vi "UHR-Fleezers Control (fpga) - 11.7.1UCBMeng3.vi"() -> ()   [LabVIEW 2014]
doc: "UHR-Fleezers Instrument Control Code (fpga)"
uses:
  <vilib>/Platform/TimedLoop/XDataNode/timing_clust.ctl
  <vilib>/Platform/TimedLoop/XDataNode/nitl_modes.ctl
  <vilib>/Platform/TimedLoop/XDataNode/wakeup.ctl
  <vilib>/rvi/Emulation/niFpgaGetClockAttributes.vi
  <vilib>/rvi/Emulation/niFpgaSctlEmulationGetInTimedLoop.vi
  <vilib>/rvi/Emulation/niFpgaEmulationReportErrorSimple.vi
  <vilib>/rvi/Emulation/niFpgaProcessEmulError.vi
  <vilib>/rvi/eio/common/nirviEmuTemplateMethod_errors.vi
  <vilib>/rvi/Emulation/niFpgaCriticalErrorInLSC.vi
  <vilib>/rvi/interface/RandomDataEmulation/niFpgaRandomDataHandleErrors.vi
  <vilib>/eio/EIONode/EIONode.xnode
  <vilib>/eio/EIOMethodNode/EIOMethodNode.xnode
  <vilib>/rvi/DataTransferAndStorage/Container/XNode/niFpgaContainer.xnode
  <vilib>/rvi/interface/RandomDataEmulation/nirviRandomDataFpgaReadWriteTemplate.vi
  <vilib>/addons/control/pid/fpga.llb/XNode/niFpgaPID.xnode
  <vilib>/Platform/TimedLoop/XDataNode/XDataNode.xnode
  <vilib>/Platform/TimedLoop/XDataNode/XDNodeRunTimeDep.lvlib
panel:
  in  "Tab Control":T1(tab)=enum."Force FB"
  in  "Set 3":bool
  in  "Set 2":bool=TRUE
  in  "Set 1":bool=TRUE
  in  "Trap Pos to FIFO":bool
  in  "N of AI1 Int Acq Sets":i16=2 min=1 max=3 step=1
  out "AI Late Counter":u8
  in  "ai count":u16=400
  in  "+ phase":bool
  in  "Phase count adjustment":i16
  out "Relative phase":i16
  in  "AI to FIFO":bool
  out "BD1 Frequency Out 1":u64
  out "BD1 Frequency Out 2":u64
  out "Trap Pos FIFO Timeout":u16
  out "Trap AI FIFO Timeout":u16
  in  "Trap FIFO Set Timeout":i32
  in  "Tab Control 2":T2(tab)
  in  "RD":bool
  in  "FB1 output high":i16=3000
  in  "FB1 output low":i16
  in  "D1":i16
  in  "I1":i16=5
  in  "P1":i16=10
  in  "Swap F1 and F2":bool
  in  "Cont. Scan":bool
  in  "Abort scan":bool
  in  "Cycles per step":u64
  in  "Scan BD":bool
  in  "Number of scans":u16
  in  "Scan steps":u64
  in  "Scan freq.  increment":i64
  out "Scanning":bool
  in  "Start scan":bool
  in  "OSK Bd 1":bool
  in  "Reset Bd 1":bool
  in  "PMODE":bool
  in  "Direct RF Box \nCommunication":bool
  in  "Data BD 2":u8 format="%08b"
  in  "Data BD 1":u8 format="%08b"
  in  "Address":u8 format="%02x"
  in  "Update Data":bool
  in  "FPGA Controls\n RF Box":bool
  in  "Number Interlace Cycles":u8=2 min=1 max=3
  in  "Interlace Off Parameters":u8=1 min=1 max=3
  in  "Interlace ON/OFF":bool
  out "DIO Relative phase":i16
  in  "Phase count adjustment (DIO)":i16
  in  "+ phase (DIO)":bool
  out "DIO Late Counter":u8
  in  "DIO count 1 (ticks)":u16=400
  in  "DIO count 2 (ticks)":u16=400
  in  "DIO count 3 (ticks)":u16=400
  out "AI2 Y Sum Set 2":i16
  out "AI2 Y Sum Set 1":i16
  in  "FB Setpoint Set 1":i16 min=0 step=1
  in  "FB Reset Set 1":bool
  in  "FB On/Off Set 1":bool
  in  "FB Reset Set 2":bool
  in  "FB On/Off Set 2":bool
  in  "FB Setpoint Set 2":i16 min=0 step=1
  out "Scan I":u64
  in  "Amp switch delay":u8=5
  in  "XY phase ext loop method":bool
  in  "BD 2 Amplitude 1":u16
  in  "BD 1 Amplitude 1":u16
  in  "BD 2 Frequency 1":u64
  in  "BD 1 Frequency 1":u64
  in  "BD 2 Amplitude 2":u16
  in  "BD 1 Amplitude 2":u16
  in  "BD 2 Frequency 2":u64
  in  "BD 1 Frequency 2":u64
  in  "BD 2 Amplitude 3":u16
  in  "BD 1 Amplitude 3":u16
  in  "BD 2 Frequency 3":u64
  in  "BD 1 Frequency 3":u64
  in  "BD 1 Delay (ticks)":u8
  in  "BD 2 Delay (Ticks)":u8 caption="Count(Ticks)"
  in  "Next trap write delay (ticks)":u8 caption="Count(Ticks)"
  in  "Trap 1 osc enable":bool
  in  "Trap 2 osc enable":bool
  in  "FB2 output high":fxp<+/-,16,1>=0.999969482421875
  in  "FB2 output low":fxp<+/-,16,1>=-1.0
  in  "P2":fxp<+/-,16,8> format="%.11g"
  in  "I2":fxp<+/-,16,8>=10.0 format="%.11g"
  in  "D2":fxp<+/-,16,8> format="%.11g"
  in  "Negate Diff?":bool
  in  "Diff FB Measurement?":bool
  in  "FB Trig Integrate":u32=1
  out "TTrig?":bool
  in  "TTrig Negate Pos":bool=TRUE
  out "Trap Pos FB Int Signal":fxp<+/-,24,9> format="%.18g"
  out "Trap Pos FB Int-Norm Signal":fxp<+/-,16,1> format="%.16g"
  in  "FPGA TTrig Thresh":i64
  in  "FPGA Trap Trig":bool
  out "Trap Pos FB Action":i64
  in  "Trap Pos. FB Offset Factor":i64
  in  "Trap Pos. FB Mult Factor":i64=2
  in  "Trap Pos. FB Reset":bool
  in  "Trap Pos FB Monitor T1 or T2":bool
  in  "AI1 X Scale":u16
  in  "Trap Pos FB Int Count":u16=100
  in  "Trap Pos FB Negate Action":bool
  out "AI1 X Set 2":fxp<+/-,16,1>
  out "AI1 X Set 1":fxp<+/-,16,1>
  in  "Trap Pos. FB SP":fxp<+/-,16,1>
  in  "Force feedback":bool
  out "TTrig Sig":i64
  out "TTrig Fin Thresh":i64
  in  "1D or 2D Scan?":bool
  in  "Abort scan (MCL)":bool
  in  "MCL Scan Axis":bool
  in  "Cont. Scan (MCL)":bool
  out "Scan I (MCL)":u64
  in  "Number of scans (MCL)":u16
  out "Scanning MCL":bool
  in  "Scan steps (MCL)":u64
  in  "Cycles per step (MCL)":u64
  in  "Scan freq.  increment (MCL)":i16
  in  "Start scan (MCL)":bool
  in  "AO2":i16
  in  "AO1":i16
  out "MCL Late Counter":u8
  in  "MCL count":u32=800
  out "MCL Relative Phase":i16
  in  "Phase count adjustment (MCL)":i16
  in  "+ phase (MCL)":bool
  out "APD2 int gate":bool
  out "APD3 out state":bool
  in  "APD Gate Operating Mode":u8 max=2 step=1
  in  "Invert APD Gate":bool
  in  "APD Gate OFF Count":u16=100
  in  "APD Gate ON Count":u16=300
  out "APD 1 Gate Late Counter":u8
  out "APD 1 Gate Relative Phase":i16
  in  "Phase count adjustment (APD 1 Gate)":i16
  in  "+ phase (APD 1 Gate)":bool
  out "APD 2 Counts 0":u32
  out "APD 2 Counts 1":u32
  out "APD 1 Counts 0":u32
  out "APD 1 Counts 1":u32
  out "APD1 out state":bool
  in  "APD AO scale factor":i16=1
  in  "APD to FIFO":bool
  in  "APD Acq Rate Count":u32=20000000
  out "APD Acq Late Counter":u8
  out "APD Acq Relative Phase":i16
  in  "Phase Count Adjustment (APD Acq)":i16
  in  "+ phase (APD Acq)":bool
  in  "Phase count adjustment (APD 2 Gate)":i16
  out "APD 2 Gate Late Counter":u8
  out "APD 2 Gate Relative Phase":i16
  in  "+ phase (APD 2 Gate)":bool
  out "APD2 out state":bool
  out "APD 3 Counts 0":u32
  out "APD 3 Counts 1":u32
  out "APD 3 Gate Late Counter":u8
  in  "Phase count adjustment (APD 3 Gate)":i16
  out "APD 3 Gate Relative Phase":i16
  in  "+ phase (APD 3 Gate)":bool
  out "APD1 int gate":bool
  out "APD3 int gate":bool
  in  "D3":i16
  in  "I3":i16=5
  in  "P3":i16=10
  in  "Green Filter Flipper":bool
  in  "Green FB Count":u16=1200
  out "Green Late Counter":u8
  out "Green FB Relative Phase":i16
  in  "Phase count adjustment (Green FB)":i16=10
  in  "+ phase (Green FB)":bool
  out "Green FB Sum":i16
  in  "Green int current ON count adj":u16=150
  in  "Current Out":u16=30000
  in  "Green FB On/Off":bool
  in  "Green FB Setpoint":i16=250 min=0 step=1
  in  "Green FB Reset":bool
  in  "Operating Mode 2":u8=2 max=2 step=1
  in  "Invert GI 2":bool
  in  "Green interlace OFF count 2":u16=900
  in  "Green interlace ON count 2":u16=300
  out "GI Late Counter 2":u8
  out "GI Relative phase 2":i16
  in  "Phase count adjustment (GI) 2":i16=20
  in  "+ phase (GI) 2":bool
  in  "Green interlace OFF count":u16=100
  out "GI Relative phase":i16
  in  "Phase count adjustment (GI)":i16
  in  "+ phase (GI)":bool
  in  "Green interlace ON count":u16=300
  out "GI Late Counter":u8
  in  "Invert GI":bool
  in  "Operating Mode":u8 max=2 step=1
  in  "+ phase (RI)":bool
  out "RI Relative phase":i16
  out "RI Late Counter":u8
  in  "Red interlace ON count":u16=300
  in  "Red interlace OFF count":u16=100
  in  "Invert RI":bool
  in  "Red Laser Operating Mode":u8 max=2 step=1
  in  "Phase count adjustment (RI)":i16
  out "Red FB Intensity":i16
  in  "RI Current Out":u16=30000
  in  "Red FB On/Off":bool
  in  "D4":i16
  in  "I4":i16=5
  in  "P4":i16=10
  in  "Red FB Setpoint":i16=250 min=0 step=1
  in  "Red FB Reset":bool
  in  "RI Operating Mode 2":u8=2 max=2 step=1
  in  "Invert RI 2":bool
  in  "Phase count adjustment (BI AO)":i16=20
  in  "Blue current ON count adj (AO)":u16=150
  in  "BI Current Out":i16=30000
  in  "Blue FB On/Off":bool
  in  "D5":i16
  in  "I5":i16=5
  in  "P5":i16=10
  in  "Blue FB Setpoint":i16=250 min=0 step=1
  in  "Blue FB Reset":bool
  in  "BI Operating Mode (AO)":u8=2 max=2 step=1
  in  "Invert BI (AO)":bool
  in  "Blue OFF count (AO)":u16=900
  in  "Blue ON count (AO)":u16=300
  out "BI Late Counter (AO)":u8
  out "BI Relative phase (AO)":i16
  in  "+ phase (BI AO)":bool
  in  "Phase count adjustment (BI D)":i16
  in  "Blue Laser Operating Mode (D)":u8 max=2 step=1
  in  "Invert BI (D)":bool
  in  "Blue interlace OFF count (D)":u16=100
  in  "Blue interlace ON count (D)":u16=300
  out "Blue Late Counter (D)":u8
  out "BI Relative phase (D)":i16
  in  "+ phase (BI D)":bool
  out "Blue Intensity":i16
  # "Only one of these can be on\nat a time:"
  # "Raster Scan AOD"
  # "1 (X)"
  # "2 (Y)"
  # "IR Intensity Feedback (RF BD 1)"
  # "FB Gains Set 1"
  # "FB output range 1"
  # "False is usual, True is external loop method"
  # "Parameters if using the external RF switching loop"
  # "Parameters if using the usual internal RF switching method"
  # "FB Triggering Excitation Laser"
  # "Trap Pos. FB Gains"
  # "Trap Pos. FB Range"
  # "AO1 (Y)"
  # "2D"
  # "1D"
  # "AO2 (X)"
  # "APD AO for aligning"
  # "Detection Loop"
  # "Green fluorescent laser digital gate interlacing loop"
  # "0 Forced ON\n1 Forced OFF\n2 Interlacing"
  # "Green FB Gains"
  # "Red fluorescent laser digital gate interlacing loop"
  # "Detection Loop"
  # "0 Forced ON\n1 Forced OFF\n2 Interlacing"
  # "Analog/FB Control Loop\n(Disabled)"
  # "Digital Control Loop"
  # "Blue laser intensity reading"
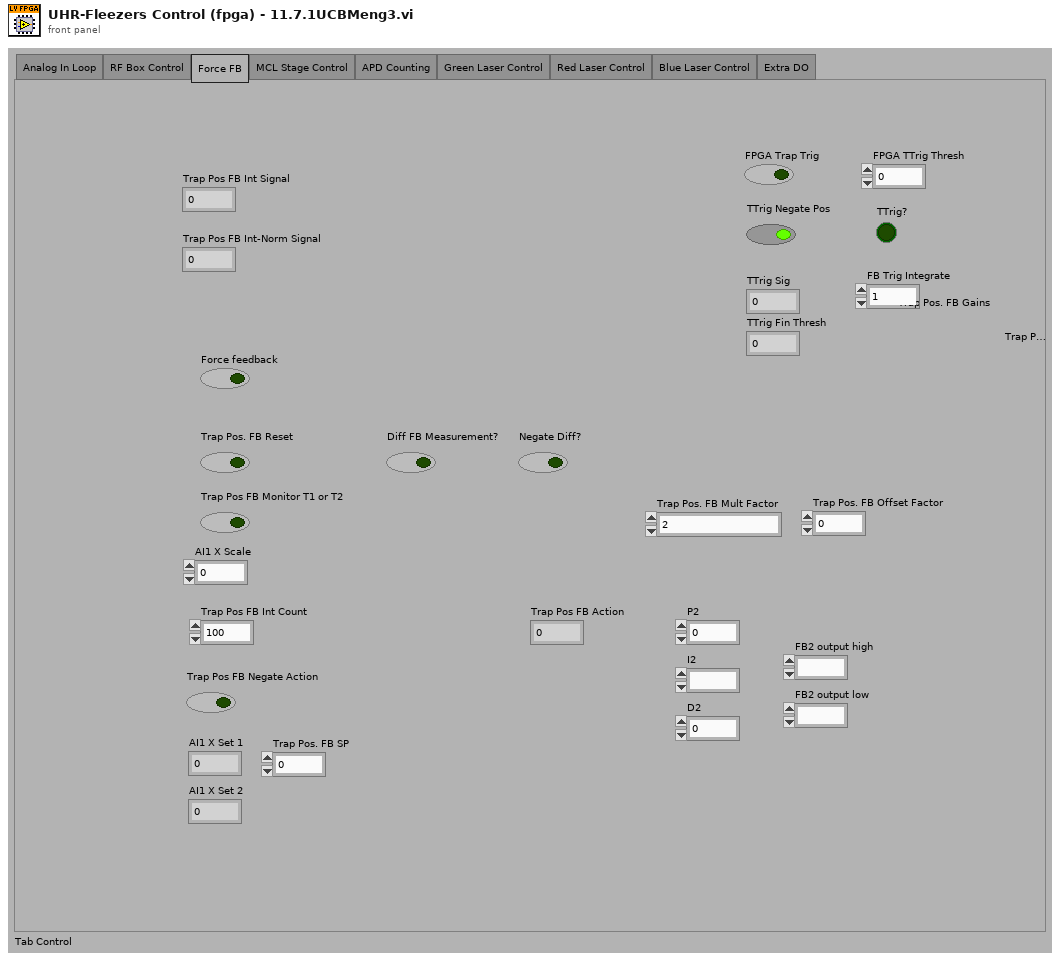
[diagram p1: front panel]
types:
  T1 = enum32{"Analog In Loop", "RF Box Control", "Force FB", "MCL Stage Control", "APD Counting", "Green Laser Control", "Red Laser Control", "Blue Laser Control", "Extra DO"}
  T2 = enum32{"Controls", "Interlacing Frequency and Amplitude Values", "Oscillate trap from memory"}
  T3 = typedef "XDNodeRunTimeDep.lvlib/timing_clust.ctl" = cluster{"Expected End [f-1]":u64, "Actual End [f-1]":u64, "Finished Late? [f-1]":bool, "Expected End [i-1]":u64, "Actual End [i-1]":u64, "Finished Late? [i-1]":bool, "Expected Start [i]":u64, "Actual Start [i]":u64, "Expected Start [f]":u64, "Actual Start [f]":u64, "Source Name":string, "Structure Name":string, "Period":i64, "Deadline":i64, "Offset":i64, "Start":i64, "Priority":i32, "Timeout":i32, "Mode":T4, "Wakeup Reason":T5, "Error":errorcluster, "Source Type":string, "Secondary Source Type":string, "Global End Time":u64, "Global Start Time":u64, "Frame Duration":u64, "Iteration Duration":u64, "Assigned CPU":i32, "I/O Scan Engine Mode":u32}
  T4 = typedef "XDNodeRunTimeDep.lvlib/nitl_modes.ctl" = enum32{"No Change", "Process missed periods, maintain original phase", "Discard missed periods, maintain original phase", "Process missed periods, ignore original phase", "Discard missed periods, ignore original phase"}
  T5 = typedef "XDNodeRunTimeDep.lvlib/wakeup.ctl" = enum32{"Normal", "Aborted", "Asynchronous wakeup", "Timing source error", "Timed loop error", "Timeout"}
  T6 = cluster{"proportional gain (Kc)":i16, "integral gain (Kc*Ts/Ti)":i16, "derivative gain (Kc*Td/Ts)":i16}
  T7 = cluster{"FB1 output high":i16, "FB1 output low":i16}
  T8 = cluster{"P2":fxp<+/-,16,8>, "I2":fxp<+/-,16,8>, "D2":fxp<+/-,16,8>}
  T9 = cluster{"FB2 output high":fxp<+/-,16,1>, "FB2 output low":fxp<+/-,16,1>}
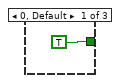
[diagram p3: hidden frame]
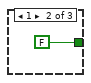
[diagram p4: hidden frame]
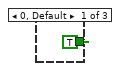
[diagram p5: hidden frame]
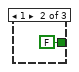
[diagram p6: hidden frame]
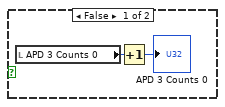
[diagram p8: hidden frame]
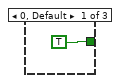
[diagram p9: hidden frame]
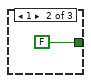
[diagram p10: hidden frame]
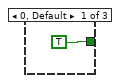
[diagram p11: hidden frame]
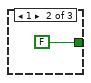
[diagram p12: hidden frame]
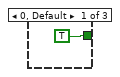
[diagram p13: hidden frame]
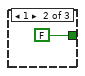
[diagram p14: hidden frame]
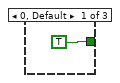
[diagram p15: hidden frame]
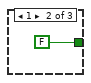
[diagram p16: hidden frame]
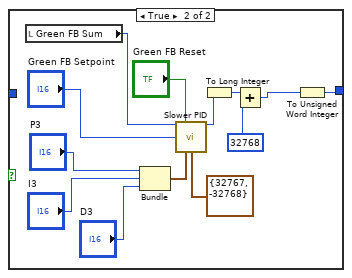
[diagram p18: hidden frame]
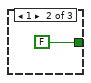
[diagram p19: hidden frame]
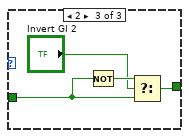
[diagram p20: hidden frame]
diagram:
  w3 = u16 0
  w5 = FALSE
  w2 = FALSE
  # "timing array current index"
  # "timing array"
  # "timing counter (phase adjusted here)"
  # "late counter"
  n1 = flat-sequence "FPGA initialization to do before running any of the loops" {
    tunnel: [u16 0 ("DIO count 3 (ticks)")] -> w1
    tunnel: [w13] -> _
    frame #0 {
      w12 = FALSE ("Enable")
      # "BD 2 (Y)"
      # "BD 1 (X)"
      # "Start up expansion chassis early\nto avoid delays later"
      # "This pin controls udclk on the RF boards.\nWhen initially configuring the boards, this pin needs to be\nconfigured as a high impedance input.  Later it will be switched\nto an output."
      # "Initial setting of DIO data and \naddress to low (before reset).  \nThis needs to happen before the other\ncontrol method loops execute."
      n2 = xnode "FPGA I/O Node"("Chassis2/Mod1/AO0"=u16 0 ("Chassis2/Mod4/AO0")) -> ("Chassis2/Mod2/AI0"=w13:i16)  [unwired: 2 in, 2 out]
      n3 = xnode "FPGA I/O Method Node"("Enable"=w12) -> ()  [unwired: 1 in, 1 out]
      n4 = xnode "FPGA I/O Method Node"("Enable"=w12) -> ()  [unwired: 1 in, 1 out]
      n5 = xnode "FPGA I/O Node"("Connector1/DIO0"=FALSE, "Connector1/DIO1"=FALSE, "Connector1/DIO2"=FALSE, "Connector1/DIO3"=FALSE, "Connector1/DIO4"=FALSE, "Connector1/DIO5"=FALSE, "Connector1/DIO6"=FALSE, "Connector1/DIO7"=FALSE, "Connector1/DIO8"=FALSE, "Connector1/DIO9"=FALSE, "Connector1/DIO10"=FALSE, "Connector1/DIO11"=FALSE, "Connector1/DIO12"=FALSE, "Connector1/DIO13"=FALSE, "Connector1/DIO15"=FALSE, "Connector1/DIO20"=FALSE, "Connector1/DIO21"=FALSE, "Connector1/DIO22"=FALSE, "Connector1/DIO23"=FALSE, "Connector1/DIO24"=FALSE, "Connector1/DIO25"=FALSE, "Connector1/DIO26"=FALSE, "Connector1/DIO27"=FALSE, "Connector1/DIO14"=FALSE) -> ()  [unwired: 24 in, 24 out]
    }
  }
  n6 = local read "AO1"() -> (w10:i16)
  n7 = local read "AO2"() -> (w9:i16)
  n8 = node-c288() -> (w8:T3)  [unwired: 1 in]
  n9 = To Unsigned Long Integer(number=w1) -> (unsigned 32bit integer=w6:u32)
  n10 = timed-loop "RF box board DIO control: control bits" {
    timing: w8 -> [_]
    timing-out: [_] -> w7
    tunnel: [w42] -> _
    tunnel: w1 -> [w42]
    stop <- FALSE stop-if-true
    n11 = xnode "FPGA I/O Node"("Connector1/DIO16"="RD", "Connector1/DIO17"="PMODE", "Connector1/DIO18"="OSK Bd 1", "Connector1/DIO19"="Reset Bd 1", "Connector0/DIO3"="Green Filter Flipper") -> ()  [unwired: 5 in, 5 out]
  }
  n12 = while "RF box board direct communication loop" {
    tunnel: w1 -> [_]
    stop <- FALSE stop-if-true
    n13 = case "Whether to use direct communication method (only use one method at a time)" shown="True" "Direct RF Box \nCommunication" {
      frame False {
      }
      frame True {
        n14 = case shown="True" "Update Data" {
          frame False {
          }
          frame True {
            n15 = flat-sequence {
              frame #0 {
                n16 = First Call?() -> (First Call?: T/F=w52:bool)
                n17 = case shown="True" w52 {
                  frame False {
                  }
                  frame True {
                    # "If first time data updated, be sure to set WR high\nbefore setting data and address bits."
                    n18 = flat-sequence {
                      frame #0 {
                        n19 = xnode "FPGA I/O Node"("Connector1/DIO15"=TRUE) -> ()  [unwired: 1 in, 1 out]
                      }
                      frame #1 {
                        n20 = call "Wait"("Count(Ticks)"=u8 40 ("DO Delay 3 (Ticks)")) -> ()  [unwired: 1 out]
                      }
                    }
                  }
                }
              }
              frame #1 {
                n21 = Number To Boolean Array(number="Address") -> (Boolean array=w101:bool[])
                n22 = Number To Boolean Array(number="Data BD 1") -> (Boolean array=w102:bool[])
                n23 = Number To Boolean Array(number="Data BD 2") -> (Boolean array=w71:bool[])
                n24 = Index Array(array=w102, index=7) -> (element=w86:bool)
                n25 = Index Array(array=w102, index=6) -> (element=w85:bool)
                n26 = Index Array(array=w102, index=5) -> (element=w84:bool)
                n27 = Index Array(array=w102, index=4) -> (element=w83:bool)
                n28 = Index Array(array=w102, index=3) -> (element=w82:bool)
                n29 = Index Array(array=w102, index=2) -> (element=w81:bool)
                n30 = Index Array(array=w102, index=1) -> (element=w80:bool)
                n31 = Index Array(array=w102, index=0) -> (element=w79:bool)
                n32 = Index Array(array=w101, index=5) -> (element=w78:bool)
                n33 = Index Array(array=w101, index=4) -> (element=w77:bool)
                n34 = Index Array(array=w101, index=3) -> (element=w76:bool)
                n35 = Index Array(array=w101, index=2) -> (element=w75:bool)
                n36 = Index Array(array=w101, index=1) -> (element=w74:bool)
                n37 = Index Array(array=w101, index=0) -> (element=w73:bool)
                n38 = Index Array(array=w71, index=7) -> (element=w62:bool)
                n39 = Index Array(array=w71, index=6) -> (element=w61:bool)
                n40 = Index Array(array=w71, index=5) -> (element=w60:bool)
                n41 = Index Array(array=w71, index=4) -> (element=w59:bool)
                n42 = Index Array(array=w71, index=3) -> (element=w58:bool)
                n43 = Index Array(array=w71, index=2) -> (element=w57:bool)
                n44 = Index Array(array=w71, index=1) -> (element=w56:bool)
                n45 = Index Array(array=w71, index=0) -> (element=w55:bool)
                n46 = xnode "FPGA I/O Node"("Connector1/DIO0"=w86, "Connector1/DIO1"=w85, "Connector1/DIO2"=w84, "Connector1/DIO3"=w83, "Connector1/DIO4"=w82, "Connector1/DIO5"=w81, "Connector1/DIO6"=w80, "Connector1/DIO7"=w79, "Connector1/DIO8"=w78, "Connector1/DIO9"=w77, "Connector1/DIO10"=w76, "Connector1/DIO11"=w75, "Connector1/DIO12"=w74, "Connector1/DIO13"=w73, "Connector1/DIO20"=w62, "Connector1/DIO21"=w61, "Connector1/DIO22"=w60, "Connector1/DIO23"=w59, "Connector1/DIO24"=w58, "Connector1/DIO25"=w57, "Connector1/DIO26"=w56, "Connector1/DIO27"=w55) -> ()  [unwired: 22 in, 22 out]
              }
              frame #2 {
                # "wait and then apply write signal"
                n47 = call "Wait2"("Count(Ticks)"=u8 40 ("DO Delay 1 (Ticks)")) -> ()  [unwired: 1 out]
              }
              frame #3 {
                # "sending bit low writes data to board buffer"
                n48 = xnode "FPGA I/O Node"("Connector1/DIO15"=FALSE) -> ()  [unwired: 1 in, 1 out]
              }
              frame #4 {
                # "wait then return write signal"
                n49 = call "Wait3"("Count(Ticks)"=u8 40 ("DO Delay 2 (Ticks)")) -> ()  [unwired: 1 out]
              }
              frame #5 {
                # "sending bit high makes ready to\nwrite more data"
                n50 = xnode "FPGA I/O Node"("Connector1/DIO15"=TRUE) -> ()  [unwired: 1 in, 1 out]
              }
            }
          }
        }
      }
    }
  }
  n51 = while "RF box board DIO control: parallel communication" {
    shift-right: [w115] -> _
    shift-left: w1 -> [w114]
    shift-right: [w113] -> _
    shift-left: FALSE ("Swap F1 and F2") -> [w112]
    stop <- FALSE stop-if-true
    n52 = flat-sequence {
      tunnel: w112 -> [w119]
      tunnel: w114 -> [w117]
      tunnel: [w119] -> w111
      tunnel: [w118] -> w110
      tunnel: [w117] -> w109
      tunnel: [w125] -> w115
      tunnel: [w124] -> w113
      tunnel: w111 -> [w123]
      tunnel: w110 -> [w121]
      tunnel: w109 -> [w120]
      frame #0 {
        n53 = call "Loop Timer"("Count(Ticks)"=w117) -> ("Tick Count(Ticks)"=w118:u16)
      }
      frame #1 {
        n54 = flat-sequence {
          tunnel: ["FPGA Controls\n RF Box"] -> w122
          tunnel: w123 -> [w126]
          tunnel: [w179] -> w125
          tunnel: [w192] -> w124
          tunnel: w122 -> [w191]
          tunnel: w121 -> [w185]
          tunnel: w120 -> [w182]
          frame #0 {
            n55 = case shown="True" "FPGA Controls\n RF Box" {
              tunnel: w126 -> [_ w128]
              frame False {
              }
              frame True {
                n56 = flat-sequence {
                  tunnel: w128 -> [w138]
                  frame #0 {
                    n57 = First Call?() -> (First Call?: T/F=w129:bool)
                    n58 = case shown="True" w129 {
                      frame False {
                      }
                      frame True {
                        # "BD 2"
                        # "BD 1"
                        # "If first time data updated, be sure to set WR high and UDCLK low\nbefore setting data and address bits."
                        n59 = xnode "FPGA I/O Method Node"("Enable"=TRUE) -> ("FPGA I/O Out"=w131:refnum<k21>)  [unwired: 1 in]
                        n60 = xnode "FPGA I/O Method Node"("Enable"=TRUE) -> ("FPGA I/O Out"=w134:refnum<k21>)  [unwired: 1 in]
                        n61 = xnode "FPGA I/O Node"("Connector1/DIO15"=TRUE) -> ()  [unwired: 1 in, 1 out]
                        n62 = xnode "FPGA I/O Node"("I/O Item"=FALSE ("Connector1/DIO30"), "FPGA I/O In"=w131) -> ()  [unwired: 1 out]
                        n63 = xnode "FPGA I/O Node"("I/O Item"=FALSE ("Connector1/DIO30"), "FPGA I/O In"=w134) -> ()  [unwired: 1 out]
                      }
                    }
                  }
                  frame #1 {
                    n64 = case shown="False" FALSE {
                      tunnel: w138 -> [w140 _]
                      frame False {
                        # "Usual operation"
                        n65 = flat-sequence "BD 1 (X)" {
                          tunnel: w140 -> [w147]
                          tunnel: "Amp switch delay" -> [w148]
                          frame #0 {
                            n66 = call "Wait6"("Count(Ticks)"="BD 1 Delay (ticks)") -> ()  [unwired: 1 out]
                          }
                          frame #1 {
                            # "switch frequency"
                            n67 = xnode "FPGA I/O Node"("Connector1/DIO36"=w147) -> ()  [unwired: 1 in, 1 out]
                          }
                          frame #2 {
                            # "~5 ticks is usual"
                            n68 = call "Wait4"("Count(Ticks)"=w148) -> ()  [unwired: 1 out]
                          }
                          frame #3 {
                            # "this switches amplitude"
                            # "switch amplitude"
                            # "send udclk high"
                            n69 = xnode "FPGA I/O Node"("Connector1/DIO30"=TRUE ("Connector1/DIO15")) -> ()  [unwired: 1 in, 1 out]
                          }
                          frame #4 {
                            # "reset to be ready for next\ncycle"
                            # "send udclk low"
                            n70 = xnode "FPGA I/O Node"("Connector1/DIO30"=FALSE ("Connector1/DIO15")) -> ()  [unwired: 1 in, 1 out]
                          }
                        }
                        n71 = flat-sequence "BD 2 (Y)" {
                          tunnel: w140 -> [w142]
                          tunnel: "Amp switch delay" -> [w143]
                          frame #0 {
                            n72 = call "Wait7"("Count(Ticks)"="BD 2 Delay (Ticks)") -> ()  [unwired: 1 out]
                          }
                          frame #1 {
                            # "switch frequency"
                            n73 = xnode "FPGA I/O Node"("Connector1/DIO37"=w142) -> ()  [unwired: 1 in, 1 out]
                          }
                          frame #2 {
                            # "~5 ticks is usual"
                            n74 = call "Wait5"("Count(Ticks)"=w143) -> ()  [unwired: 1 out]
                          }
                          frame #3 {
                            # "this switches amplitude"
                            # "switch amplitude"
                            # "send udclk high"
                            n75 = xnode "FPGA I/O Node"("Connector1/DIO29"=TRUE ("Connector1/DIO15")) -> ()  [unwired: 1 in, 1 out]
                          }
                          frame #4 {
                            # "reset to be ready for next\ncycle"
                            # "send udclk low"
                            n76 = xnode "FPGA I/O Node"("Connector1/DIO29"=FALSE ("Connector1/DIO15")) -> ()  [unwired: 1 in, 1 out]
                          }
                        }
                      }
                      frame True {
                        # "Operation when you need a long delay for either X or Y to synchonize AOD light out phase (> ~100 ticks)."
                        # "Trigger the external loop by sending the boolean FSK value through a FIFO"
                      }
                    }
                  }
                }
              }
            }
          }
          frame #1 {
            # "This is the prior cycle's on time"
            # "increment timing\nindex, reset to 0 if \nend of matrix"
            # "Reset to begginning (1) when number of cycles reached."
            # "timing index"
            # "build byte stacks for writing data\n(must correspond to addresses array constant)"
            # "Timing housekeeping"
            # "Adjust phase if late\n(maintains constant phase relationship between cycles)"
            n77 = Bundle("FB1 output high"="FB1 output high", "FB1 output low"="FB1 output low") -> (w152:T7)  [unwired: 1 in]
            n78 = Bundle("P1"="P1", "I1"="I1", "D1"="D1") -> (w153:cluster{"P1":i16, "I1":i16, "D1":i16})  [unwired: 1 in]
            n79 = feedback #1(u8 0 ("t")) -> (w188:u8)
            n80 = Increment(x=w188) -> (x+1=w231:u8)
            n81 = Increment(x="Number Interlace Cycles") -> (x+1=w226:u8)
            n82 = Equal?(x=w231, y=w226) -> (x = y?=w233:bool)
            n83 = Select(t=u8 1, s=w233, f=w231) -> (s? t:f=w187:u8)
            n84 = feedback-in #1(w187) -> ()
            n85 = Increment(x=w187) -> (x+1=w228:u8)
            n86 = Equal?(x=w228, y=w226) -> (x = y?=w229:bool)
            n87 = Select(t=u8 1, s=w229, f=w228) -> (s? t:f=w225:u8)
            n88 = Select(t=w225, s="Interlace ON/OFF", f="Interlace Off Parameters") -> (s? t:f=w151:u8)
            n89 = case shown="2" w151 {
              tunnel: [w311 w467 "BD 1 Frequency 3"] -> w221
              tunnel: [w310 "BD 2 Frequency 2" "BD 2 Frequency 3"] -> w210
              tunnel: ["BD 2 Amplitude 1" "BD 2 Amplitude 2" "BD 2 Amplitude 3"] -> w167
              tunnel: [w299 w472 "BD 1 Amplitude 3"] -> w170
              tunnel: w153 -> [w273 w469 _]
              tunnel: w152 -> [w274 w468 _]
              frame 1, Default {
                w290 = fxp<+/-,24,9> 0.0 ("AI1 X Set 2")
                w283 = u16 0
                w306 = u64 0 ("f")
                # "This signal integration happens no matter what\nso that correct setpoints can be chosen before \nturning on the FB."
                # "Trap 1"
                n90 = local read "AI1 X Set 2"() -> (w286:fxp<+/-,16,1>)
                n91 = local read "AI1 X Set 1"() -> (w287:fxp<+/-,16,1>)
                n92 = local read "Scanning"() -> (w312:bool)
                n93 = Or(x=w312, y="Start scan") -> (x .or. y?=w304:bool)
                n94 = case shown="False" "Diff FB Measurement?" {
                  tunnel: w286 -> [w320 w329]
                  tunnel: w287 -> [w319 w330]
                  tunnel: [w317 w321] -> w288
                  frame False {
                    n95 = Select(t=w319, s="Trap Pos FB Monitor T1 or T2", f=w320) -> (s? t:f=w317:fxp<+/-,16,1>)
                  }
                  frame True {
                    n96 = Subtract(x=w330, y=w329) -> (x-y=w322:fxp<+/-,17,2>)
                    n97 = Not(x="Negate Diff?") -> (.not. x?=w328:bool)
                    n98 = Boolean To (0,1)(Boolean="Negate Diff?") -> (0, 1=w326:i16)
                    n99 = Boolean To (0,1)(Boolean=w328) -> (0, 1=w327:i16)
                    n100 = Negate(x=w326) -> (-x=w325:i16)
                    n101 = Add(x=w325, y=w327) -> (x+y=w323:i16)
                    n102 = Multiply(x=w323, y=w322) -> (x*y=w321:fxp<+/-,32,17>)
                  }
                }
                n103 = Not(x="Abort scan") -> (.not. x?=w302:bool)
                n104 = And(x=w302, y=w304) -> (x .and. y?=w301:bool)
                n105 = case "For raster scanning" shown="True" w301 {
                  tunnel: [u64 0 w456] -> w307
                  tunnel: "Start scan" -> [_ w441]
                  frame False {
                    n106 = local write "Scanning"(FALSE ("scanning")) -> ()
                  }
                  frame True {
                    w425 = i64 0
                    w424 = u64 0
                    # "scan incr."
                    # "freq. incr. mult."
                    # "count steps"
                    # "count number of cycles"
                    n107 = feedback #2(w424) -> (w453:u64)
                    n108 = Select(t=w424, s=w441, f=w453) -> (s? t:f=w455:u64)
                    n109 = Increment(x=w455) -> (x+1=w452:u64)
                    n110 = Greater?(x="Cycles per step", y=w452) -> (0:w434:bool)
                    n111 = Select(t=w452, s=w434, f=w424) -> (s? t:f=w451:u64)
                    n112 = feedback-in #2(w451) -> ()
                    n113 = feedback #3(w424) -> (w450:u64)
                    n114 = Select(t=w424, s=w441, f=w450) -> (s? t:f=w445:u64)
                    n115 = Increment(x=w445) -> (x+1=w449:u64)
                    n116 = Add(x="Scan steps", y="Scan steps") -> (x+y=w448:u64)
                    n117 = Select(t=w445, s=w434, f=w449) -> (s? t:f=w429:u64)
                    n118 = Greater?(x=w448, y=w429) -> (0:w428:bool)
                    n119 = Select(t=w429, s=w428, f=w424) -> (s? t:f=w446:u64)
                    n120 = feedback-in #3(w446) -> ()
                    n121 = Equal?(x="Scan steps", y=w429) -> (x = y?=w433:bool)
                    n122 = Greater?(x="Scan steps", y=w445) -> (0:w444:bool)
                    n123 = feedback #4(w425) -> (w447:i64)
                    n124 = Select(t=w425, s=w441, f=w447) -> (s? t:f=w431:i64)
                    n125 = Increment(x=w431) -> (x+1=w443:i64)
                    n126 = Decrement(x=w431) -> (x-1=w442:i64)
                    n127 = Select(t=w443, s=w444, f=w442) -> (s? t:f=w432:i64)
                    n128 = Select(t=w431, s=w433, f=w432) -> (s? t:f=w430:i64)
                    n129 = Select(t=w431, s=w434, f=w430) -> (s? t:f=w426:i64)
                    n130 = Select(t=w426, s=w428, f=w425) -> (s? t:f=w427:i64)
                    n131 = feedback-in #4(w427) -> ()
                    n132 = feedback #5(w424) -> (w440:u64)
                    n133 = Select(t=w424, s=w441, f=w440) -> (s? t:f=w436:u64)
                    n134 = Increment(x=w436) -> (x+1=w437:u64)
                    n135 = Select(t=w436, s=w428, f=w437) -> (s? t:f=w435:u64)
                    n136 = Greater?(x="Number of scans", y=w435) -> (0:w421:bool)
                    n137 = Multiply(x="Scan freq.  increment", y=w431) -> (x*y=w456:i64)
                    n138 = Select(t=TRUE, s="Cont. Scan", f=w421) -> (s? t:f=w420:bool)
                    "Scanning" <- w420
                    n139 = Select(t=w435, s=w420, f=w424) -> (s? t:f=w438:u64)
                    n140 = feedback-in #5(w438) -> ()
                    n141 = Increment(x=w435) -> (x+1=→"Scan I":u64)
                  }
                }
                n142 = feedback #6(w283) -> (w282:u16)
                n143 = Increment(x=w282) -> (x+1=w284:u16)
                n144 = Greater Or Equal?(x=w284, y="Trap Pos FB Int Count") -> (x >= y?=w275:bool)
                n145 = Select(t=w283, s=w275, f=w284) -> (s? t:f=w285:u16)
                n146 = feedback-in #6(w285) -> ()
                n147 = feedback #7(w290) -> (w289:fxp<+/-,24,9>)
                n148 = Add(x=w288, y=w289) -> (x+y=w281:fxp<+/-,24,9>)
                n149 = case "For intensity feedback" shown="True" "FB On/Off Set 1" {
                  tunnel: "BD 1 Amplitude 1" -> [w458 _]
                  tunnel: [w458 w462] -> w299
                  tunnel: w274 -> [_ w459]
                  tunnel: w273 -> [_ w460]
                  frame False {
                  }
                  frame True {
                    n150 = local read "AI2 Y Sum Set 1"() -> (w463:i16)
                    n151 = call "Slower PID.vi"("process variable"=w463, "reset?"="FB Reset Set 1", "setpoint"="FB Setpoint Set 1", "PID gains (x 2^8)"=w460, "output range"=w459) -> ("output"=w464:i16)  [unwired: 10 out]
                    n152 = To Unsigned Word Integer(number=w464) -> (unsigned 16bit integer=w462:u16)
                  }
                }
                n153 = Select(t=w290, s=w275, f=w281) -> (s? t:f=w293:fxp<+/-,24,9>)
                n154 = feedback-in #7(w293) -> ()
                n155 = Divide(x=w281, y="Trap Pos FB Int Count") -> (x/y=w276:fxp<+/-,16,1>)
                n156 = feedback #8(fxp<+/-,24,9> 0.0 ("AI1 X Set 2")) -> (w294:fxp<+/-,24,9>)
                n157 = Select(t=w281, s=w275, f=w294) -> (s? t:f=w295:fxp<+/-,24,9>)
                "Trap Pos FB Int Signal" <- w295
                n158 = feedback-in #8(w295) -> ()
                n159 = feedback #9(fxp<+/-,16,1> 0.0 ("Trap Pos FB Int-Norm Signal")) -> (w278:fxp<+/-,16,1>)
                n160 = Select(t=w276, s=w275, f=w278) -> (s? t:f=w277:fxp<+/-,16,1>)
                "Trap Pos FB Int-Norm Signal" <- w277
                n161 = feedback-in #9(w277) -> ()
                n162 = case "For position feedback" shown="True" "Force feedback" {
                  tunnel: [i64 0 w336] -> w296
                  tunnel: w276 -> [_ w333]
                  tunnel: w275 -> [_ w332]
                  frame False {
                  }
                  frame True {
                    n163 = feedback #10(i64 0) -> (w335:i64)
                    n164 = case shown="True" w332 {
                      tunnel: [w337 w351] -> w336
                      tunnel: w335 -> [w337 _]
                      tunnel: w333 -> [_ w345]
                      frame False {
                      }
                      frame True {
                        w355 = u32 0
                        n165 = Bundle("P2"="P2", "I2"="I2", "D2"="D2") -> (w341:T8)  [unwired: 1 in]
                        n166 = Bundle("FB2 output high"="FB2 output high", "FB2 output low"="FB2 output low") -> (w338:T9)  [unwired: 1 in]
                        n167 = xnode ("PID")("process variable"=w345, "reset?"="Trap Pos. FB Reset", "setpoint"="Trap Pos. FB SP", "PID gains"=w341, "output range"=w338) -> ("output"=w367:fxp<+/-,16,1>)
                        n168 = Negate(x=w367) -> (-x=w366:fxp<+/-,17,2>)
                        n169 = Select(t=w366, s="Trap Pos FB Negate Action", f=w367) -> (s? t:f=w363:fxp<+/-,17,2>)
                        n170 = Scale By Power Of 2(n=u32 15, x=u32 1) -> (x*2^n=w360:u32)
                        n171 = Multiply(x=w363, y=w360) -> (x*y=w359:fxp<+/-,17,17>)
                        n172 = To Quad Integer(1:w359) -> (0:w371:i64)
                        "Trap Pos FB Action" <- w371
                        n173 = Multiply(x=w371, y="Trap Pos. FB Mult Factor") -> (x*y=w369:i64)
                        n174 = Add(x=w369, y="Trap Pos. FB Offset Factor") -> (x+y=w351:i64)
                        n175 = feedback #11() -> (w352:i64)  [unwired: 1 in]
                        n176 = Add(x=w351, y=w352) -> (x+y=w349:i64)
                        n177 = feedback #12(w355) -> (w357:u32)
                        n178 = Increment(x=w357) -> (x+1=w346:u32)
                        n179 = Greater Or Equal?(x=w346, y="FB Trig Integrate") -> (x >= y?=w347:bool)
                        n180 = Select(t=i64 0, s=w347, f=w349) -> (s? t:f=w353:i64)
                        n181 = feedback-in #11(w353) -> ()
                        n182 = Select(t=w355, s=w347, f=w346) -> (s? t:f=w356:u32)
                        n183 = feedback-in #12(w356) -> ()
                        n184 = And(x=w347, y="FPGA Trap Trig") -> (x .and. y?=w354:bool)
                        n185 = case "Trap FB trigger excitation laser ON" shown="True" w354 {
                          tunnel: w349 -> [_ w375]
                          tunnel: w346 -> [_ w373]
                          frame False {
                          }
                          frame True {
                            n186 = Not(x="TTrig Negate Pos") -> (.not. x?=w382:bool)
                            n187 = Boolean To (0,1)(Boolean="TTrig Negate Pos") -> (0, 1=w380:i16)
                            n188 = Boolean To (0,1)(Boolean=w382) -> (0, 1=w381:i16)
                            n189 = Negate(x=w380) -> (-x=w379:i16)
                            n190 = Add(x=w379, y=w381) -> (x+y=w378:i16)
                            n191 = Multiply(x=w378, y=w375) -> (x*y=w377:i64)
                            "TTrig Sig" <- w377
                            n192 = Multiply(x="FPGA TTrig Thresh", y=w373) -> (x*y=w374:i64)
                            "TTrig Fin Thresh" <- w374
                            n193 = Greater Or Equal?(x=w377, y=w374) -> (x >= y?=w376:bool)
                            n194 = case shown="True" w376 {
                              frame False {
                              }
                              frame True {
                                w385 = TRUE ("Green FB On/Off")
                                w387 = u8 2 ("Operating Mode")
                                n195 = local write "Operating Mode 2"(w387) -> ()
                                n196 = local write "Operating Mode"(w387) -> ()
                                n197 = local write "Green FB On/Off"(w385) -> ()
                                n198 = local write "FPGA Trap Trig"(FALSE ("FPGA Trap Trig")) -> ()
                                "TTrig?" <- w385
                              }
                            }
                          }
                        }
                      }
                    }
                    n199 = feedback-in #10(w336) -> ()
                  }
                }
                n200 = Select(t=w306, s="Scan BD", f=w307) -> (s? t:f=w305:u64)
                n201 = Select(t=w307, s="Scan BD", f=w306) -> (s? t:f=w308:u64)
                n202 = Add(x=w305, y="BD 2 Frequency 1") -> (x+y=w310:u64)
                n203 = Compound Arithmetic op=ADD(i64 0 ("f"), "BD 1 Frequency 1", w296, w308) -> (w311:u64)
                "BD1 Frequency Out 1" <- w311
              }
              frame 2 {
                # "Trap 2"
                n204 = case shown="True" "FB On/Off Set 2" {
                  tunnel: [w476 w479] -> w472
                  tunnel: "BD 1 Amplitude 2" -> [w476 _]
                  tunnel: w469 -> [_ w478]
                  tunnel: w468 -> [_ w477]
                  frame False {
                  }
                  frame True {
                    n205 = local read "AI2 Y Sum Set 2"() -> (w482:i16)
                    n206 = call "Slower PID.vi"("process variable"=w482, "reset?"="FB Reset Set 2", "setpoint"="FB Setpoint Set 2", "PID gains (x 2^8)"=w478, "output range"=w477) -> ("output"=w480:i16)  [unwired: 10 out]
                    n207 = To Unsigned Word Integer(number=w480) -> (unsigned 16bit integer=w479:u16)
                  }
                }
                n208 = Add(x="BD 1 Frequency 2", y=i64 0 ("f")) -> (x+y=w467:u64)
                "BD1 Frequency Out 2" <- w467
              }
              frame 3 {
                # "Fluorescence period"
              }
            }
            n209 = feedback-in #13(w185) -> ()
            n210 = feedback #13(w185) -> (w184:u16)
            n211 = Select(t=w187, s="Interlace ON/OFF", f="Interlace Off Parameters") -> (s? t:f=w224:u8)
            n212 = Subtract(x=w185, y=w184) -> (x-y=w183:u16)
            n213 = Subtract "The error"(x=w183, y=w182) -> (x-y=w160:u16)
            n214 = case shown="1, Default" w224 {
              tunnel: ["DIO count 1 (ticks)" "DIO count 2 (ticks)" "DIO count 3 (ticks)"] -> w181
              frame 1, Default {
              }
              frame 2 {
              }
              frame 3 {
              }
            }
            n215 = Number To Boolean Array(number=w160) -> (Boolean array=w161:bool[])
            n216 = Or Array Elements(Boolean array=w161) -> (logical OR=w159:bool)
            n217 = Boolean To (0,1)(Boolean=w159) -> (0, 1=w166:i16)
            n218 = To Unsigned Byte Integer(number=w166) -> (unsigned 8bit integer=w163:u8)
            n219 = feedback #14(u8 0) -> (w164:u8)
            n220 = Add(x=w163, y=w164) -> (x+y=w162:u8)
            "DIO Late Counter" <- w162
            n221 = feedback-in #14(w162) -> ()
            n222 = Subtract(x=w181, y=w160) -> (x-y=w180:u16)
            n223 = Split Number(x=w221) -> (hi(x)=w220:u32, lo(x)=w219:u32)
            n224 = Split Number(x=w210) -> (hi(x)=w215:u32, lo(x)=w214:u32)
            n225 = Boolean To (0,1)(Boolean="+ phase (DIO)") -> (0, 1=w177:i16)
            n226 = Split Number(x=w220) -> (lo(x)=w218:u16)  [unwired: 1 out]
            n227 = Split Number(x=w219) -> (hi(x)=w217:u16, lo(x)=w216:u16)
            n228 = Split Number(x=w215) -> (lo(x)=w213:u16)  [unwired: 1 out]
            n229 = Split Number(x=w214) -> (hi(x)=w212:u16, lo(x)=w211:u16)
            n230 = Split Number(x=w170) -> (hi(x)=w172:u8, lo(x)=w171:u8)
            n231 = Split Number(x=w167) -> (hi(x)=w169:u8, lo(x)=w168:u8)
            n232 = Split Number(x=w218) -> (hi(x)=w209:u8, lo(x)=w208:u8)
            n233 = Split Number(x=w217) -> (hi(x)=w207:u8, lo(x)=w206:u8)
            n234 = Split Number(x=w213) -> (hi(x)=w202:u8, lo(x)=w201:u8)
            n235 = Split Number(x=w216) -> (hi(x)=w205:u8, lo(x)=w204:u8)
            n236 = Split Number(x=w212) -> (hi(x)=w200:u8, lo(x)=w199:u8)
            n237 = Split Number(x=w211) -> (hi(x)=w198:u8, lo(x)=w197:u8)
            n238 = Multiply(x=w177, y="Phase count adjustment (DIO)") -> (x*y=w173:i16)
            n239 = feedback #15(i16 0) -> (w175:i16)
            n240 = Subtract(x=w175, y=w173) -> (x-y=w174:i16)
            "DIO Relative phase" <- w174
            n241 = feedback-in #15(w174) -> ()
            n242 = Add(x=w180, y=w173) -> (x+y=w179:u16)
            n243 = Build Array "BD 1 A Stack"(w172, w171) -> (w194:u8[])
            n244 = Build Array "BD 2 A Stack"(w169, w168) -> (w193:u8[])
            n245 = Build Array "BD 1 nu Stack"(w209, w208, w207, w206, w205, w204) -> (w203:u8[])
            n246 = Build Array "BD 2 nu Stack"(w202, w201, w200, w199, w198, w197) -> (w196:u8[])
            n247 = case shown="2" w151 {
              tunnel: [w264 w267] -> w192
              tunnel: [u8 10 u8 4] -> w195
              tunnel: "Swap F1 and F2" -> [w265 w267]
              frame 2 {
                # "F2"
                n248 = Not(x=w265) -> (.not. x?=w264:bool)
              }
              frame 1, Default {
                # "low chooses F1"
                # "F1"
              }
            }
            n249 = case "If FPGA is controlling (toggling) RF synth" shown="True" w191 {
              tunnel: w203 -> [_ w240]
              tunnel: w196 -> [_ w239]
              tunnel: w195 -> [_ w238]
              tunnel: w194 -> [_ w237]
              tunnel: w193 -> [_ w236]
              frame False {
              }
              frame True {
                # "Write next amp.\n(wait until beginning of next loop iteration to update)"
                n250 = flat-sequence "Update the next F1 and F2 frequency value (the actual frequency won't change until FSK is switched).\nThen load the next amplitude value into buffer, but don't update it until the next cycle." {
                  tunnel: w239 -> [w242]
                  tunnel: w240 -> [w243]
                  tunnel: [w243] -> w235
                  tunnel: [w242] -> w234
                  tunnel: w238 -> [w244]
                  tunnel: w235 -> [w246]
                  tunnel: w234 -> [w245]
                  tunnel: w237 -> [w257]
                  tunnel: w236 -> [w256]
                  frame #0 {
                    # "To possibly send\nthese writes to very\nend of loop (for x and\ny phase adjust)"
                    n251 = call "Wait8"("Count(Ticks)"="Next trap write delay (ticks)") -> ()  [unwired: 1 out]
                  }
                  frame #1 {
                    n252 = for {
                      tunnel: w246 -> [w252] mode=indexing
                      tunnel: w245 -> [w251] mode=indexing
                      tunnel: w244 -> [w249]
                      i -> [w250]
                      # "Write next freq."
                      n253 = To Unsigned Byte Integer(number=w250) -> (unsigned 8bit integer=w247:u8)
                      n254 = Add(x=w249, y=w247) -> (x+y=w248:u8)
                      n255 = call "write to RF synth bd.vi"("Address Byte"=w248, "BD 2 Byte"=w251, "BD 1 Byte"=w252) -> ()
                    }
                  }
                  frame #2 {
                    w253 = TRUE ("Connector1/DIO15")
                    # "send udclk high\n(BD 1 and 2)"
                    n256 = xnode "FPGA I/O Node"("Connector1/DIO30"=w253, "Connector1/DIO29"=w253) -> ()  [unwired: 2 in, 2 out]
                  }
                  frame #3 {
                    w254 = FALSE ("Connector1/DIO15")
                    n257 = xnode "FPGA I/O Node"("Connector1/DIO30"=w254, "Connector1/DIO29"=w254) -> ()  [unwired: 2 in, 2 out]
                  }
                  frame #4 {
                    n258 = for {
                      tunnel: w257 -> [w263] mode=indexing
                      tunnel: w256 -> [w262] mode=indexing
                      tunnel: u8 33 -> [w260]
                      i -> [w261]
                      n259 = To Unsigned Byte Integer(number=w261) -> (unsigned 8bit integer=w258:u8)
                      n260 = Add(x=w260, y=w258) -> (x+y=w259:u8)
                      n261 = call "write to RF synth bd.vi"("Address Byte"=w259, "BD 2 Byte"=w262, "BD 1 Byte"=w263) -> ()
                    }
                  }
                }
              }
            }
          }
        }
      }
    }
  }
  n262 = while "APD 1 Counter" {
    tunnel: w1 -> [_]
    stop <- FALSE stop-if-true
    n263 = flat-sequence {
      frame #0 {
        n264 = xnode "FPGA I/O Method Node"("FPGA I/O In"=refnum<k21> "Connector0/DIO0" ("APD 1 DO"), "Timeout"=-1) -> ()  [unwired: 2 out]
      }
      frame #1 {
        n265 = local read "APD1 int gate"() -> (w491:bool)
        n266 = case shown="True" w491 {
          frame False {
          }
          frame True {
            n267 = local read "APD1 out state"() -> (w492:bool)
            n268 = case shown="True" w492 {
              frame False {
                n269 = local read "APD 1 Counts 0"() -> (w494:u32)
                n270 = Increment(x=w494) -> (x+1=→"APD 1 Counts 0":u32)
              }
              frame True {
                n271 = local read "APD 1 Counts 1"() -> (w496:u32)
                n272 = Increment(x=w496) -> (x+1=→"APD 1 Counts 1":u32)
              }
            }
          }
        }
      }
    }
  }
  n273 = while "APD 2 Counter" {
    tunnel: w1 -> [_]
    stop <- FALSE stop-if-true
    n274 = flat-sequence {
      frame #0 {
        n275 = xnode "FPGA I/O Method Node"("FPGA I/O In"=refnum<k21> "Connector0/DIO1" ("APD 2 DO"), "Timeout"=-1) -> ()  [unwired: 2 out]
      }
      frame #1 {
        n276 = local read "APD2 int gate"() -> (w500:bool)
        n277 = case shown="True" w500 {
          frame False {
          }
          frame True {
            n278 = local read "APD2 out state"() -> (w501:bool)
            n279 = case shown="False" w501 {
              frame False {
                n280 = local read "APD 2 Counts 0"() -> (w503:u32)
                n281 = Increment(x=w503) -> (x+1=→"APD 2 Counts 0":u32)
              }
              frame True {
                n282 = local read "APD 2 Counts 1"() -> (w505:u32)
                n283 = Increment(x=w505) -> (x+1=→"APD 2 Counts 1":u32)
              }
            }
          }
        }
      }
    }
  }
  n284 = while "APD 2 Gating" {
    shift-right: [w509] -> _
    shift-left: w1 -> [w514]
    shift-right: [w508] -> _
    shift-left: w5 -> [w506]
    stop <- FALSE stop-if-true
    n285 = flat-sequence {
      tunnel: w514 -> [w517]
      tunnel: [w518] -> w512
      tunnel: [w517] -> w510
      tunnel: [w516] -> w507
      tunnel: w506 -> [w516]
      tunnel: [w521] -> w513
      tunnel: w512 -> [w521]
      tunnel: [w520] -> w511
      tunnel: w510 -> [w520]
      tunnel: w507 -> [w519]
      tunnel: [w543] -> w509
      tunnel: w513 -> [w553]
      tunnel: w511 -> [w551]
      tunnel: [w522] -> w508
      frame #0 {
        n286 = call "Loop Timer8"("Count(Ticks)"=w517) -> ("Tick Count(Ticks)"=w518:u16)
      }
      frame #1 {
        # "Signal maybe then sent through \na transistor before APD"
        n287 = xnode "FPGA I/O Node"("Connector0/DIO8"=w519, "Connector0/DIO9"=w519, "Connector0/DIO10"=w519, "Connector0/DIO11"=w519) -> ()  [unwired: 4 in, 4 out]
        "APD2 int gate" <- w519
      }
      frame #2 {
        n288 = local read "APD Gate ON Count"() -> (w536:u16)
        n289 = local read "APD Gate OFF Count"() -> (w535:u16)
        n290 = feedback #16(TRUE) -> (w548:bool)
        n291 = feedback-in #17(w553) -> ()
        n292 = feedback #17(w553) -> (w537:u16)
        n293 = Not(x=w548) -> (.not. x?=w546:bool)
        n294 = feedback-in #16(w546) -> ()
        n295 = Subtract(x=w553, y=w537) -> (x-y=w552:u16)
        n296 = Select(t=w536, s=w546, f=w535) -> (s? t:f=w550:u16)
        n297 = Subtract(x=w552, y=w551) -> (x-y=w528:u16)
        n298 = Subtract(x=w550, y=w528) -> (x-y=w542:u16)
        n299 = Number To Boolean Array(number=w528) -> (Boolean array=w527:bool[])
        n300 = Or Array Elements(Boolean array=w527) -> (logical OR=w526:bool)
        n301 = Boolean To (0,1)(Boolean="+ phase (APD 2 Gate)") -> (0, 1=w540:i16)
        n302 = Multiply(x=w540, y="Phase count adjustment (APD 2 Gate)") -> (x*y=w538:i16)
        n303 = Boolean To (0,1)(Boolean=w526) -> (0, 1=w533:i16)
        n304 = Add(x=w542, y=w538) -> (x+y=w543:u16)
        n305 = To Unsigned Byte Integer(number=w533) -> (unsigned 8bit integer=w530:u8)
        n306 = feedback #18(i16 0) -> (w545:i16)
        n307 = Subtract(x=w545, y=w538) -> (x-y=w544:i16)
        "APD 2 Gate Relative Phase" <- w544
        n308 = feedback-in #18(w544) -> ()
        n309 = feedback #19(u8 0) -> (w531:u8)
        n310 = Add(x=w530, y=w531) -> (x+y=w529:u8)
        "APD 2 Gate Late Counter" <- w529
        n311 = feedback-in #19(w529) -> ()
        n312 = local read "APD Gate Operating Mode"() -> (w534:u8)
        n313 = case shown="2" w534 {
          tunnel: [TRUE FALSE w556] -> w523
          tunnel: w548 -> [_ _ w556]
          frame 0, Default {
          }
          frame 1 {
          }
          frame 2 {
          }
        }
        n314 = local read "Invert APD Gate"() -> (w525:bool)
        n315 = Not(x=w523) -> (.not. x?=w524:bool)
        n316 = Select(t=w524, s=w525, f=w523) -> (s? t:f=w522:bool)
      }
    }
  }
  n317 = while "532 nm green fluorescent laser interlacing (DO to IA 532 nm AOM ME amp)." {
    shift-right: [w560] -> _
    shift-left: w1 -> [w565]
    shift-right: [w559] -> _
    shift-left: w2 -> [w557]
    stop <- FALSE stop-if-true
    n318 = flat-sequence {
      tunnel: w565 -> [w568]
      tunnel: [w569] -> w563
      tunnel: [w568] -> w561
      tunnel: [w567] -> w558
      tunnel: w557 -> [w567]
      tunnel: [w572] -> w564
      tunnel: w563 -> [w572]
      tunnel: [w571] -> w562
      tunnel: w561 -> [w571]
      tunnel: w558 -> [w570]
      tunnel: [w581] -> w560
      tunnel: w564 -> [w601]
      tunnel: w562 -> [w598]
      tunnel: [w590] -> w559
      frame #0 {
        n319 = call "Loop Timer4"("Count(Ticks)"=w568) -> ("Tick Count(Ticks)"=w569:u16)
      }
      frame #1 {
        n320 = xnode "FPGA I/O Node"("Connector1/DIO34"=w570, "Connector1/DIO38"=w570, "Connector1/DIO39"=w570) -> ()  [unwired: 3 in, 3 out]
      }
      frame #2 {
        n321 = feedback-in #20(w601) -> ()
        n322 = feedback #20(w601) -> (w600:u16)
        n323 = Subtract(x=w601, y=w600) -> (x-y=w599:u16)
        n324 = Subtract(x=w599, y=w598) -> (x-y=w574:u16)
        n325 = Number To Boolean Array(number=w574) -> (Boolean array=w575:bool[])
        n326 = Or Array Elements(Boolean array=w575) -> (logical OR=w573:bool)
        n327 = Boolean To (0,1)(Boolean="+ phase (GI)") -> (0, 1=w586:i16)
        n328 = Multiply(x=w586, y="Phase count adjustment (GI)") -> (x*y=w583:i16)
        n329 = Boolean To (0,1)(Boolean=w573) -> (0, 1=w580:i16)
        n330 = To Unsigned Byte Integer(number=w580) -> (unsigned 8bit integer=w577:u8)
        n331 = feedback #21(i16 0) -> (w584:i16)
        n332 = feedback #22(u8 0) -> (w578:u8)
        n333 = Add(x=w577, y=w578) -> (x+y=w576:u8)
        "GI Late Counter" <- w576
        n334 = feedback-in #22(w576) -> ()
        n335 = Subtract(x=w584, y=w583) -> (x-y=w582:i16)
        "GI Relative phase" <- w582
        n336 = feedback-in #21(w582) -> ()
        n337 = feedback #23(TRUE) -> (w593:bool)
        n338 = case shown="2" "Operating Mode" {
          tunnel: [TRUE FALSE w607] -> w590
          tunnel: w593 -> [_ _ w604]
          frame 0, Default {
          }
          frame 1 {
          }
          frame 2 {
            n339 = Not(x=w604) -> (.not. x?=w606:bool)
            n340 = Select(t=w606, s="Invert GI", f=w604) -> (s? t:f=w607:bool)
          }
        }
        n341 = Not(x=w593) -> (.not. x?=w589:bool)
        n342 = Select(t="Green interlace ON count", s=w589, f="Green interlace OFF count") -> (s? t:f=w595:u16)
        n343 = Subtract(x=w595, y=w574) -> (x-y=w587:u16)
        n344 = Add(x=w587, y=w583) -> (x+y=w581:u16)
        n345 = feedback-in #23(w589) -> ()
      }
    }
  }
  n346 = while "Green and red fluorescent laser interlacing (Current AO to IA 532 nm AOM ME amp)." {
    shift-right: [w616] -> _
    shift-left: w1 -> [w619]
    shift-right: [w613] -> _
    shift-left: w3 -> [w611]
    shift-right: [w610] -> _
    shift-left: w3 -> [w609]
    stop <- FALSE stop-if-true
    n347 = flat-sequence {
      tunnel: w619 -> [w623]
      tunnel: [w624] -> w618
      tunnel: [w623] -> w617
      tunnel: [w622] -> w612
      tunnel: w611 -> [w622]
      tunnel: w609 -> [w621]
      tunnel: [w621] -> w608
      tunnel: [w628] -> w615
      tunnel: w618 -> [w628]
      tunnel: [w627] -> w614
      tunnel: w617 -> [w627]
      tunnel: w612 -> [w626]
      tunnel: w608 -> [w625]
      tunnel: [w649] -> w616
      tunnel: [w665] -> w613
      tunnel: w615 -> [w676]
      tunnel: w614 -> [w673]
      tunnel: [w633] -> w610
      frame #0 {
        n348 = call "Loop Timer10"("Count(Ticks)"=w623) -> ("Tick Count(Ticks)"=w624:u16)
      }
      frame #1 {
        n349 = xnode "FPGA I/O Node"("Chassis2/Mod1/AO0"=w626, "Chassis2/Mod1/AO1"=w625) -> ()  [unwired: 2 in, 2 out]
      }
      frame #2 {
        # "Design note:\n\nThese two laser controls are in the same loop\nbecause the expansion current AI cannot separately\ntime the outputs fast enough for us.  Apparently\nit is because of communication time between the\nexpansion card and the fpga.\n\nSo the two analog control signals have the same timing\nand profile, but independent amplitudes to independently\ncontrol the intensity and feedback for each laser."
        n350 = feedback #24(TRUE) -> (w629:bool)
        n351 = Not(x=w629) -> (.not. x?=w630:bool)
        n352 = feedback-in #24(w630) -> ()
        n353 = Subtract(x="Green interlace OFF count 2", y="Green int current ON count adj") -> (x-y=w658:u16)
        n354 = feedback-in #25(w676) -> ()
        n355 = feedback #25(w676) -> (w675:u16)
        n356 = Add(x="Green int current ON count adj", y="Green interlace ON count 2") -> (x+y=w659:u16)
        n357 = Subtract(x=w676, y=w675) -> (x-y=w674:u16)
        n358 = Select(t=w659, s=w630, f=w658) -> (s? t:f=w670:u16)
        n359 = Subtract(x=w674, y=w673) -> (x-y=w642:u16)
        n360 = case shown="2" "RI Operating Mode 2" {
          tunnel: [TRUE FALSE w682] -> w631
          tunnel: w629 -> [_ _ w679]
          frame 0, Default {
          }
          frame 1 {
          }
          frame 2 {
            n361 = Not(x=w679) -> (.not. x?=w681:bool)
            n362 = Select(t=w681, s="Invert RI 2", f=w679) -> (s? t:f=w682:bool)
          }
        }
        n363 = Subtract(x=w670, y=w642) -> (x-y=w653:u16)
        n364 = case shown="0, Default" "Operating Mode 2" {
          tunnel: [TRUE FALSE w716] -> w634
          tunnel: w629 -> [_ _ w713]
          frame 0, Default {
          }
          frame 1 {
          }
          frame 2 {
            n365 = Not(x=w713) -> (.not. x?=w715:bool)
            n366 = Select(t=w715, s="Invert GI 2", f=w713) -> (s? t:f=w716:bool)
          }
        }
        n367 = Number To Boolean Array(number=w642) -> (Boolean array=w643:bool[])
        n368 = Boolean To (0,1)(Boolean="+ phase (GI) 2") -> (0, 1=w655:i16)
        n369 = Or Array Elements(Boolean array=w643) -> (logical OR=w641:bool)
        n370 = Boolean To (0,1)(Boolean=w641) -> (0, 1=w648:i16)
        n371 = Multiply(x=w655, y="Phase count adjustment (GI) 2") -> (x*y=w651:i16)
        n372 = To Unsigned Byte Integer(number=w648) -> (unsigned 8bit integer=w644:u8)
        n373 = Add(x=w653, y=w651) -> (x+y=w649:u16)
        n374 = feedback #26(u8 0) -> (w646:u8)
        n375 = Add(x=w644, y=w646) -> (x+y=w645:u8)
        "GI Late Counter 2" <- w645
        n376 = feedback-in #26(w645) -> ()
        n377 = feedback #27(i16 0) -> (w652:i16)
        n378 = Subtract(x=w652, y=w651) -> (x-y=w650:i16)
        "GI Relative phase 2" <- w650
        n379 = feedback-in #27(w650) -> ()
        n380 = And(x=w634, y="Green FB On/Off") -> (x .and. y?=w660:bool)
        n381 = And(x=w631, y="Red FB On/Off") -> (x .and. y?=w640:bool)
        n382 = case shown="False" w660 {
          tunnel: "Current Out" -> [w697 _]
          tunnel: [w697 w706] -> w664
          frame False {
          }
          frame True {
            n383 = local read "Green FB Sum"() -> (w702:i16)
            n384 = Bundle("P3"="P3", "I3"="I3", "D3"="D3") -> (w698:cluster{"P3":i16, "I3":i16, "D3":i16})  [unwired: 1 in]
            n385 = call "Slower PID.vi"("process variable"=w702, "reset?"="Green FB Reset", "setpoint"="Green FB Setpoint", "PID gains (x 2^8)"=w698, "output range"=cluster{"output high":i16, "output low":i16} {"output high"=32767, "output low"=-32768} ("Green FB output range")) -> ("output"=w709:i16)  [unwired: 10 out]
            n386 = To Long Integer(number=w709) -> (32bit integer=w703:i32)
            n387 = Add(x=w703, y=32768) -> (x+y=w705:i32)
            n388 = To Unsigned Word Integer(number=w705) -> (unsigned 16bit integer=w706:u16)
          }
        }
        n389 = case shown="True" w640 {
          tunnel: "RI Current Out" -> [w683 _]
          tunnel: [w683 w692] -> w636
          frame False {
          }
          frame True {
            n390 = local read "Red FB Intensity"() -> (w688:i16)
            n391 = Bundle("P4"="P4", "I4"="I4", "D4"="D4") -> (w684:cluster{"P4":i16, "I4":i16, "D4":i16})  [unwired: 1 in]
            n392 = call "Slower PID.vi"("process variable"=w688, "reset?"="Red FB Reset", "setpoint"="Red FB Setpoint", "PID gains (x 2^8)"=w684, "output range"=cluster{"output high":i16, "output low":i16} {"output high"=32767, "output low"=-32768} ("Green FB output range")) -> ("output"=w695:i16)  [unwired: 10 out]
            n393 = To Long Integer(number=w695) -> (32bit integer=w689:i32)
            n394 = Add(x=w689, y=32768) -> (x+y=w691:i32)
            n395 = To Unsigned Word Integer(number=w691) -> (unsigned 16bit integer=w692:u16)
          }
        }
        n396 = Boolean To (0,1)(Boolean=w634) -> (0, 1=w666:i16)
        n397 = Boolean To (0,1)(Boolean=w631) -> (0, 1=w635:i16)
        n398 = To Unsigned Word Integer(number=w666) -> (unsigned 16bit integer=w663:u16)
        n399 = To Unsigned Word Integer(number=w635) -> (unsigned 16bit integer=w637:u16)
        n400 = Multiply(x=w663, y=w664) -> (x*y=w665:u16)
        n401 = Multiply(x=w637, y=w636) -> (x*y=w633:u16)
      }
    }
  }
  n402 = while "Excitation laser intensity feedback measurement (all lasers)" {
    shift-right: [w717] -> _
    shift-left: w1 -> [w722]
    stop <- FALSE stop-if-true
    n403 = flat-sequence {
      tunnel: w722 -> [w724]
      tunnel: [w725] -> w720
      tunnel: [w724] -> w718
      tunnel: [w731] -> w721
      tunnel: w720 -> [w731]
      tunnel: [w730] -> w719
      tunnel: w718 -> [w730]
      tunnel: [w743] -> w717
      tunnel: w721 -> [w754]
      tunnel: w719 -> [w751]
      frame #0 {
        n404 = call "Loop Timer9"("Count(Ticks)"=w724) -> ("Tick Count(Ticks)"=w725:u16)
      }
      frame #1 {
        # "Design note:\n\nAll lasers need to be measured at the same \ntime because the AI expansion module\ncannot independently time the measurements\nwithin our requirements: their is dead time.\n\nThis probably wouldn't be an issue with the built\nin AI on the fpga board itself."
        n405 = xnode "FPGA I/O Node"("Connector1/DIO35"=TRUE) -> ("Chassis2/Mod2/AI2"=→"Blue Intensity":i16, "Chassis2/Mod2/AI1"=→"Red FB Intensity":i16, "Chassis2/Mod2/AI0"=→"Green FB Sum":i16)  [unwired: 4 in, 4 out]
      }
      frame #2 {
        n406 = feedback-in #28(w754) -> ()
        n407 = feedback #28(w754) -> (w753:u16)
        n408 = Subtract(x=w754, y=w753) -> (x-y=w752:u16)
        n409 = xnode "FPGA I/O Node"("Connector1/DIO35"=FALSE) -> ()  [unwired: 1 in, 1 out]
        n410 = Subtract(x=w752, y=w751) -> (x-y=w733:u16)
        n411 = Subtract(x="Green FB Count", y=w733) -> (x-y=w747:u16)
        n412 = Number To Boolean Array(number=w733) -> (Boolean array=w734:bool[])
        n413 = Or Array Elements(Boolean array=w734) -> (logical OR=w732:bool)
        n414 = Boolean To (0,1)(Boolean="+ phase (Green FB)") -> (0, 1=w745:i16)
        n415 = Boolean To (0,1)(Boolean=w732) -> (0, 1=w739:i16)
        n416 = Multiply(x=w745, y="Phase count adjustment (Green FB)") -> (x*y=w740:i16)
        n417 = Add(x=w747, y=w740) -> (x+y=w743:u16)
        n418 = To Unsigned Byte Integer(number=w739) -> (unsigned 8bit integer=w736:u8)
        n419 = feedback #29(i16 0) -> (w742:i16)
        n420 = Subtract(x=w742, y=w740) -> (x-y=w741:i16)
        "Green FB Relative Phase" <- w741
        n421 = feedback-in #29(w741) -> ()
        n422 = feedback #30(u8 0) -> (w737:u8)
        n423 = Add(x=w736, y=w737) -> (x+y=w735:u8)
        "Green Late Counter" <- w735
        n424 = feedback-in #30(w735) -> ()
      }
    }
  }
  n425 = while "APD 1 Gating" {
    shift-right: [w758] -> _
    shift-left: w1 -> [w763]
    shift-right: [w757] -> _
    shift-left: w5 -> [w755]
    stop <- FALSE stop-if-true
    n426 = flat-sequence {
      tunnel: w763 -> [w766]
      tunnel: [w767] -> w761
      tunnel: [w766] -> w759
      tunnel: [w765] -> w756
      tunnel: w755 -> [w765]
      tunnel: [w770] -> w762
      tunnel: w761 -> [w770]
      tunnel: [w769] -> w760
      tunnel: w759 -> [w769]
      tunnel: w756 -> [w768]
      tunnel: [w788] -> w758
      tunnel: w762 -> [w802]
      tunnel: w760 -> [w799]
      tunnel: [w771] -> w757
      frame #0 {
        n427 = call "Loop Timer7"("Count(Ticks)"=w766) -> ("Tick Count(Ticks)"=w767:u16)
      }
      frame #1 {
        # "Signal maybe then sent through \na transistor before APD"
        n428 = xnode "FPGA I/O Node"("Connector0/DIO4"=w768, "Connector0/DIO5"=w768, "Connector0/DIO6"=w768, "Connector0/DIO7"=w768) -> ()  [unwired: 4 in, 4 out]
        "APD1 int gate" <- w768
      }
      frame #2 {
        n429 = feedback #31(TRUE) -> (w794:bool)
        n430 = feedback-in #32(w802) -> ()
        n431 = feedback #32(w802) -> (w801:u16)
        n432 = Not(x=w794) -> (.not. x?=w791:bool)
        n433 = feedback-in #31(w791) -> ()
        n434 = Subtract(x=w802, y=w801) -> (x-y=w800:u16)
        n435 = Select(t="APD Gate ON Count", s=w791, f="APD Gate OFF Count") -> (s? t:f=w796:u16)
        n436 = Subtract(x=w800, y=w799) -> (x-y=w776:u16)
        n437 = Subtract(x=w796, y=w776) -> (x-y=w787:u16)
        n438 = Number To Boolean Array(number=w776) -> (Boolean array=w777:bool[])
        n439 = Or Array Elements(Boolean array=w777) -> (logical OR=w775:bool)
        n440 = Boolean To (0,1)(Boolean="+ phase (APD 1 Gate)") -> (0, 1=w785:i16)
        n441 = Boolean To (0,1)(Boolean=w775) -> (0, 1=w782:i16)
        n442 = Multiply(x=w785, y="Phase count adjustment (APD 1 Gate)") -> (x*y=w783:i16)
        n443 = To Unsigned Byte Integer(number=w782) -> (unsigned 8bit integer=w779:u8)
        n444 = Add(x=w787, y=w783) -> (x+y=w788:u16)
        n445 = feedback #33(i16 0) -> (w790:i16)
        n446 = Subtract(x=w790, y=w783) -> (x-y=w789:i16)
        "APD 1 Gate Relative Phase" <- w789
        n447 = feedback-in #33(w789) -> ()
        n448 = feedback #34(u8 0) -> (w780:u8)
        n449 = Add(x=w779, y=w780) -> (x+y=w778:u8)
        "APD 1 Gate Late Counter" <- w778
        n450 = feedback-in #34(w778) -> ()
        n451 = case shown="2" "APD Gate Operating Mode" {
          tunnel: [TRUE FALSE w805] -> w772
          tunnel: w794 -> [_ _ w805]
          frame 0, Default {
          }
          frame 1 {
          }
          frame 2 {
          }
        }
        n452 = Not(x=w772) -> (.not. x?=w773:bool)
        n453 = Select(t=w773, s="Invert APD Gate", f=w772) -> (s? t:f=w771:bool)
      }
    }
  }
  n454 = while "MCL stage control" {
    shift-right: [w818] -> _
    shift-left: w1 -> [w821]
    shift-right: [w811] -> _
    shift-left: w10 -> [w808]
    shift-right: [w810] -> _
    shift-left: w9 -> [w806]
    stop <- FALSE stop-if-true
    n455 = flat-sequence {
      tunnel: w821 -> [w825]
      tunnel: [w826] -> w817
      tunnel: [w825] -> w815
      tunnel: [w824] -> w809
      tunnel: w808 -> [w824]
      tunnel: [w823] -> w807
      tunnel: w806 -> [w823]
      tunnel: w817 -> [w830]
      tunnel: [w830] -> w816
      tunnel: w815 -> [w829]
      tunnel: [w829] -> w814
      tunnel: w809 -> [w828]
      tunnel: w807 -> [w827]
      tunnel: w816 -> [w838]
      tunnel: w814 -> [w837]
      tunnel: [w838] -> w820
      tunnel: [w837] -> w819
      tunnel: [w836] -> w813
      tunnel: [w835] -> w812
      tunnel: [w910] -> w818
      tunnel: w820 -> [w917]
      tunnel: w819 -> [w914]
      tunnel: w813 -> [w912]
      tunnel: w812 -> [w911]
      tunnel: [w912] -> w811
      tunnel: [w911] -> w810
      frame #0 {
        n456 = call "Loop Timer5"("Count(Ticks)"=w825) -> ("Tick Count(Ticks)"=w826:u32)
      }
      frame #1 {
        n457 = xnode "FPGA I/O Node"("Connector0/AO1"=w828, "Connector0/AO2"=w827) -> ()  [unwired: 2 in, 2 out]
      }
      frame #2 {
        n458 = local read "Scanning MCL"() -> (w850:bool)
        n459 = Or(x=w850, y="Start scan (MCL)") -> (x .or. y?=w845:bool)
        n460 = Not(x="Abort scan (MCL)") -> (.not. x?=w843:bool)
        n461 = And(x=w843, y=w845) -> (x .and. y?=w842:bool)
        n462 = case "Raster scan" shown="True" w842 {
          tunnel: [w851 w894] -> w847
          tunnel: "Start scan (MCL)" -> [_ w879]
          tunnel: [w851 w855] -> w831
          frame False {
            w851 = i16 0
            n463 = local write "Scanning MCL"(FALSE ("scanning")) -> ()
          }
          frame True {
            w865 = i16 0
            w864 = u64 0
            # "scan incr."
            # "freq. incr. mult."
            # "count steps"
            # "count number of cycles"
            n464 = feedback #35(w864) -> (w891:u64)
            n465 = Select(t=w864, s=w879, f=w891) -> (s? t:f=w893:u64)
            n466 = Increment(x=w893) -> (x+1=w890:u64)
            n467 = Greater?(x="Cycles per step (MCL)", y=w890) -> (0:w874:bool)
            n468 = Select(t=w890, s=w874, f=w864) -> (s? t:f=w889:u64)
            n469 = feedback-in #35(w889) -> ()
            n470 = feedback #36(w864) -> (w888:u64)
            n471 = Select(t=w864, s=w879, f=w888) -> (s? t:f=w883:u64)
            n472 = Increment(x=w883) -> (x+1=w887:u64)
            n473 = Add(x="Scan steps (MCL)", y="Scan steps (MCL)") -> (x+y=w886:u64)
            n474 = Select(t=w883, s=w874, f=w887) -> (s? t:f=w869:u64)
            n475 = Greater?(x=w886, y=w869) -> (0:w868:bool)
            n476 = Select(t=w869, s=w868, f=w864) -> (s? t:f=w884:u64)
            n477 = feedback-in #36(w884) -> ()
            n478 = Equal?(x="Scan steps (MCL)", y=w869) -> (x = y?=w873:bool)
            n479 = Greater?(x="Scan steps (MCL)", y=w883) -> (0:w882:bool)
            n480 = feedback #37(w865) -> (w885:i16)
            n481 = Select(t=w865, s=w879, f=w885) -> (s? t:f=w871:i16)
            n482 = Increment(x=w871) -> (x+1=w881:i16)
            n483 = Decrement(x=w871) -> (x-1=w880:i16)
            n484 = Select(t=w881, s=w882, f=w880) -> (s? t:f=w872:i16)
            n485 = Select(t=w871, s=w873, f=w872) -> (s? t:f=w870:i16)
            n486 = Select(t=w871, s=w874, f=w870) -> (s? t:f=w866:i16)
            n487 = Select(t=w866, s=w868, f=w865) -> (s? t:f=w867:i16)
            n488 = feedback-in #37(w867) -> ()
            n489 = feedback #38(w864) -> (w878:u64)
            n490 = Select(t=w864, s=w879, f=w878) -> (s? t:f=w853:u64)
            n491 = Increment(x=w853) -> (x+1=w875:u64)
            n492 = Select(t=w853, s=w868, f=w875) -> (s? t:f=w854:u64)
            n493 = Greater?(x="Number of scans (MCL)", y=w854) -> (0:w861:bool)
            n494 = Multiply(x="Scan freq.  increment (MCL)", y=w871) -> (x*y=w894:i16)
            n495 = Select(t=TRUE, s="Cont. Scan (MCL)", f=w861) -> (s? t:f=w860:bool)
            "Scanning MCL" <- w860
            n496 = Select(t=w854, s=w860, f=w864) -> (s? t:f=w876:u64)
            n497 = feedback-in #38(w876) -> ()
            n498 = Increment(x=w854) -> (x+1=→"Scan I (MCL)":u64)
            n499 = To Word Integer(number=w853) -> (16bit integer=w856:i16)
            n500 = Multiply(x=w856, y="Scan freq.  increment (MCL)") -> (x*y=w855:i16)
          }
        }
        n501 = Select(t=w831, s="1D or 2D Scan?", f=i16 0) -> (s? t:f=w832:i16)
        n502 = Select(t=w832, s="MCL Scan Axis", f=w847) -> (s? t:f=w846:i16)
        n503 = Select(t=w847, s="MCL Scan Axis", f=w832) -> (s? t:f=w848:i16)
        n504 = Add(x=w846, y="AO2") -> (x+y=w835:i16)
        n505 = Add(x="AO1", y=w848) -> (x+y=w836:i16)
      }
      frame #3 {
        n506 = feedback-in #39(w917) -> ()
        n507 = feedback #39(w917) -> (w916:u32)
        n508 = Boolean To (0,1)(Boolean="+ phase (MCL)") -> (0, 1=w908:i16)
        n509 = Subtract(x=w917, y=w916) -> (x-y=w915:u32)
        n510 = Multiply(x=w908, y="Phase count adjustment (MCL)") -> (x*y=w904:i16)
        n511 = Subtract(x=w915, y=w914) -> (x-y=w896:u32)
        n512 = Subtract(x="MCL count", y=w896) -> (x-y=w906:u32)
        n513 = feedback #40(i16 0) -> (w905:i16)
        n514 = Subtract(x=w905, y=w904) -> (x-y=w903:i16)
        "MCL Relative Phase" <- w903
        n515 = feedback-in #40(w903) -> ()
        n516 = Number To Boolean Array(number=w896) -> (Boolean array=w897:bool[])
        n517 = Or Array Elements(Boolean array=w897) -> (logical OR=w895:bool)
        n518 = Boolean To (0,1)(Boolean=w895) -> (0, 1=w902:i16)
        n519 = Add(x=w906, y=w904) -> (x+y=w910:u32)
        n520 = To Unsigned Byte Integer(number=w902) -> (unsigned 8bit integer=w899:u8)
        n521 = feedback #41(u8 0) -> (w900:u8)
        n522 = Add(x=w899, y=w900) -> (x+y=w898:u8)
        "MCL Late Counter" <- w898
        n523 = feedback-in #41(w898) -> ()
      }
    }
  }
  n524 = while "Control APD data integration - stream to host" {
    shift-right: [w922] -> _
    shift-left: w6 -> [w927]
    stop <- FALSE stop-if-true
    n525 = flat-sequence {
      tunnel: w927 -> [w929]
      tunnel: [w930] -> w925
      tunnel: [w929] -> w923
      tunnel: [w940] -> w926
      tunnel: w925 -> [w940]
      tunnel: [w939] -> w924
      tunnel: w923 -> [w939]
      tunnel: [w938] -> w921
      tunnel: [w937] -> w920
      tunnel: [w931] -> w919
      tunnel: [w982] -> w922
      tunnel: w926 -> [w992]
      tunnel: w924 -> [w989]
      tunnel: w921 -> [w975]
      tunnel: w920 -> [w974]
      tunnel: w919 -> [w962]
      frame #0 {
        n526 = call "Loop Timer6"("Count(Ticks)"=w929) -> ("Tick Count(Ticks)"=w930:u32)
      }
      frame #1 {
        n527 = flat-sequence {
          tunnel: [w942] -> w936
          tunnel: w936 -> [w945]
          tunnel: [w949] -> w935
          tunnel: [w948] -> w934
          tunnel: [w945] -> w933
          tunnel: [w944] -> w932
          tunnel: [w956] -> w937
          tunnel: [w957] -> w938
          tunnel: w935 -> [w957]
          tunnel: w934 -> [w956]
          tunnel: w933 -> [w955]
          tunnel: w932 -> [w954]
          tunnel: [w954] -> w931
          frame #0 {
            # "use separate variable so each APD won't\nhave to wait to read"
            n528 = feedback #42(FALSE) -> (w941:bool)
            "APD1 out state" <- w941
            "APD2 out state" <- w941
            "APD3 out state" <- w941
            n529 = Not(x=w941) -> (.not. x?=w942:bool)
            n530 = feedback-in #42(w942) -> ()
          }
          frame #1 {
            n531 = local read "APD 3 Counts 1"() -> (w947:u32)
            n532 = local read "APD 3 Counts 0"() -> (w946:u32)
            n533 = local read "APD 1 Counts 1"() -> (w953:u32)
            n534 = local read "APD 1 Counts 0"() -> (w952:u32)
            n535 = local read "APD 2 Counts 1"() -> (w951:u32)
            n536 = local read "APD 2 Counts 0"() -> (w950:u32)
            n537 = Select(t=w947, s=w945, f=w946) -> (s? t:f=w944:u32)
            n538 = Select(t=w953, s=w945, f=w952) -> (s? t:f=w949:u32)
            n539 = Select(t=w951, s=w945, f=w950) -> (s? t:f=w948:u32)
          }
          frame #2 {
            n540 = case shown="False" w955 {
              frame False {
                w958 = u32 0 ("APD 1 Counts 0")
                n541 = local write "APD 1 Counts 0"(w958) -> ()
                n542 = local write "APD 2 Counts 0"(w958) -> ()
                n543 = local write "APD 3 Counts 0"(w958) -> ()
              }
              frame True {
                w959 = u32 0 ("APD 1 Counts 1")
                n544 = local write "APD 1 Counts 1"(w959) -> ()
                n545 = local write "APD 2 Counts 1"(w959) -> ()
                n546 = local write "APD 3 Counts 1"(w959) -> ()
              }
            }
          }
        }
      }
      frame #2 {
        n547 = feedback-in #43(w992) -> ()
        n548 = feedback #43(w992) -> (w991:u32)
        n549 = Subtract(x=w992, y=w991) -> (x-y=w990:u32)
        n550 = Subtract(x=w990, y=w989) -> (x-y=w967:u32)
        n551 = case shown="True" "APD to FIFO" {
          tunnel: w975 -> [_ w997]
          tunnel: w974 -> [_ w995]
          tunnel: w962 -> [_ w993]
          frame False {
          }
          frame True {
            n552 = flat-sequence {
              tunnel: 0 ("Timeout") -> [w999]
              tunnel: w997 -> [w1000]
              tunnel: [w999] -> w996
              tunnel: w996 -> [w1001]
              tunnel: w995 -> [w1002]
              tunnel: [w1001] -> w994
              tunnel: w994 -> [w1004]
              tunnel: w993 -> [w1003]
              frame #0 {
                n553 = xnode ("FIFO Write")("Element"=w1000, "Timeout"=w999) -> ()  [unwired: 1 in, 2 out]
              }
              frame #1 {
                n554 = xnode ("FIFO Write")("Element"=w1002, "Timeout"=w1001) -> ()  [unwired: 1 in, 2 out]
              }
              frame #2 {
                n555 = xnode ("FIFO Write")("Element"=w1003, "Timeout"=w1004) -> ()  [unwired: 1 in, 2 out]
              }
            }
          }
        }
        n556 = Subtract(x="APD Acq Rate Count", y=w967) -> (x-y=w983:u32)
        n557 = Number To Boolean Array(number=w967) -> (Boolean array=w968:bool[])
        n558 = Or Array Elements(Boolean array=w968) -> (logical OR=w966:bool)
        n559 = Boolean To (0,1)(Boolean=w966) -> (0, 1=w973:i16)
        n560 = To Unsigned Byte Integer(number=w973) -> (unsigned 8bit integer=w970:u8)
        n561 = feedback #44(u8 0) -> (w971:u8)
        n562 = Add(x=w970, y=w971) -> (x+y=w969:u8)
        "APD Acq Late Counter" <- w969
        n563 = feedback-in #44(w969) -> ()
        n564 = Boolean To (0,1)(Boolean="+ phase (APD Acq)") -> (0, 1=w979:i16)
        n565 = Multiply(x=w979, y="Phase Count Adjustment (APD Acq)") -> (x*y=w976:i16)
        n566 = Add(x=w983, y=w976) -> (x+y=w982:u32)
        n567 = feedback #45(i16 0) -> (w981:i16)
        n568 = Subtract(x=w981, y=w976) -> (x-y=w978:i16)
        "APD Acq Relative Phase" <- w978
        n569 = feedback-in #45(w978) -> ()
        n570 = To Word Integer(number=w975) -> (16bit integer=w984:i16)
        n571 = To Word Integer(number=w962) -> (16bit integer=w963:i16)
        n572 = To Word Integer(number=w974) -> (16bit integer=w985:i16)
        n573 = Multiply(x="APD AO scale factor", y=w985) -> (x*y=w964:i16)
        n574 = Multiply(x="APD AO scale factor", y=w963) -> (x*y=w960:i16)
        n575 = Multiply(x="APD AO scale factor", y=w984) -> (x*y=w965:i16)
        n576 = xnode "FPGA I/O Node"("Connector0/AO6"=w965, "Connector0/AO7"=w964, "Connector0/AO5"=w960) -> ()  [unwired: 3 in, 3 out]
      }
    }
  }
  n577 = while "DAQ AI set 1" {
    shift-right: [w1005] -> _
    shift-left: w1 -> [w1010]
    stop <- FALSE stop-if-true
    n578 = flat-sequence {
      tunnel: w1010 -> [w1020]
      tunnel: [w1021] -> w1008
      tunnel: [w1020] -> w1007
      tunnel: [w1031] -> w1018
      tunnel: [w1030] -> w1017
      tunnel: [w1029] -> w1016
      tunnel: [w1028] -> w1015
      tunnel: [w1027] -> w1014
      tunnel: [w1026] -> w1013
      tunnel: [w1025] -> w1012
      tunnel: [w1024] -> w1011
      tunnel: [w1023] -> w1009
      tunnel: w1008 -> [w1023]
      tunnel: w1007 -> [w1022]
      tunnel: [w1022] -> w1006
      tunnel: [w1061] -> w1005
      tunnel: w1018 -> [w1087]
      tunnel: w1017 -> [w1053]
      tunnel: w1016 -> [w1054]
      tunnel: w1015 -> [w1033]
      tunnel: w1014 -> [w1077]
      tunnel: w1013 -> [w1076]
      tunnel: w1012 -> [w1075]
      tunnel: w1011 -> [w1074]
      tunnel: w1009 -> [w1071]
      tunnel: w1006 -> [w1068]
      frame #0 {
        n579 = call "Loop Timer3"("Count(Ticks)"=w1020) -> ("Tick Count(Ticks)"=w1021:u16)
      }
      frame #1 {
        n580 = xnode "FPGA I/O Node"("Connector1/DIO31"=TRUE ("Connector1/DIO33")) -> ("Connector0/AI0"=w1031:i16, "Connector0/AI1"=w1030:i16, "Connector0/AI2"=w1029:i16, "Connector0/AI3"=w1028:i16, "Connector0/AI4"=w1027:i16, "Connector0/AI5"=w1026:i16, "Connector0/AI6"=w1025:i16, "Connector0/AI7"=w1024:i16)  [unwired: 9 in, 9 out]
      }
      frame #2 {
        w1057 = FALSE ("AI to FIFO")
        # "Adjust phase after data acquired if button pressed"
        n581 = feedback #46(i16 1) -> (w1080:i16)
        n582 = Increment(x=w1080) -> (x+1=w1086:i16)
        n583 = Scale By Power Of 2(n="AI1 X Scale", x=w1053) -> (x*2^n=w1051:i16)
        n584 = Greater?(x=w1086, y="N of AI1 Int Acq Sets") -> (0:w1083:bool)
        n585 = Select(t=i16 1, s=w1083, f=w1086) -> (s? t:f=w1085:i16)
        n586 = feedback-in #46(w1085) -> ()
        n587 = Divide(x=w1051, y=w1033) -> (x/y=w1050:fxp<+/-,16,1>)
        n588 = feedback #47(w1057) -> (w1055:bool)
        n589 = feedback #48(w1057) -> (w1073:bool)
        n590 = case shown="2" w1080 {
          tunnel: w1054 -> [w1110 w1117 _]
          tunnel: ["Set 1" "Set 2" "Set 3"] -> w1078
          tunnel: ["AI to FIFO" w1119 w1124] -> w1072
          tunnel: w1073 -> [_ w1119 w1124]
          tunnel: ["Trap Pos to FIFO" w1118 w1123] -> w1056
          tunnel: w1055 -> [_ w1118 w1123]
          tunnel: w1050 -> [w1109 w1116 _]
          tunnel: [w1108 w1114 FALSE] -> w1037
          tunnel: [w1107 w1115 u64 0 ("BD1 Frequency Out 2")] -> w1036
          frame 1, Default {
            n591 = local read "BD1 Frequency Out 1"() -> (w1107:u64)
            n592 = Compound Arithmetic op=AND("Trap Pos to FIFO", "Set 1", "AI to FIFO") -> (w1108:bool)
            "AI2 Y Sum Set 1" <- w1110
            "AI1 X Set 1" <- w1109
          }
          frame 2 {
            n593 = local read "BD1 Frequency Out 2"() -> (w1115:u64)
            n594 = Compound Arithmetic op=AND(w1118, "Set 2", w1119) -> (w1114:bool)
            "AI2 Y Sum Set 2" <- w1117
            "AI1 X Set 2" <- w1116
          }
          frame 3 {
          }
        }
        n595 = And(x=w1078, y=w1072) -> (x .and. y?=w1079:bool)
        n596 = case shown="True" w1079 {
          tunnel: w1087 -> [_ w1138]
          tunnel: w1053 -> [_ w1137]
          tunnel: w1054 -> [_ w1136]
          tunnel: w1033 -> [_ w1135]
          tunnel: w1077 -> [_ w1134]
          tunnel: w1076 -> [_ w1133]
          tunnel: w1075 -> [_ w1132]
          tunnel: w1074 -> [_ w1131]
          tunnel: 0 ("DMA buffer timeout") -> [_ w1140]
          frame False {
          }
          frame True {
            n597 = Build Array(w1138, w1137, w1136, w1135, w1134, w1133, w1132, w1131) -> (w1139:i16[])
            n598 = for {
              tunnel: w1139 -> [w1142] mode=indexing
              tunnel: w1140 -> [w1143]
              tunnel: [w1141] -> w1129 mode=indexing
              n599 = xnode ("FIFO Write")("Element"=w1142, "Timeout"=w1143) -> ("Timed Out?"=w1141:bool)  [unwired: 1 in, 1 out]
            }
            n600 = Or Array Elements(Boolean array=w1129) -> (logical OR=w1126:bool)
            n601 = Boolean To (0,1)(Boolean=w1126) -> (0, 1=w1128:i16)
            n602 = feedback #49(u16 0) -> (w1127:u16)
            n603 = Add(x=w1128, y=w1127) -> (x+y=w1125:u16)
            "Trap AI FIFO Timeout" <- w1125
            n604 = feedback-in #49(w1125) -> ()
          }
        }
        n605 = feedback-in #47(w1056) -> ()
        n606 = feedback-in #48(w1072) -> ()
        n607 = case shown="True" w1037 {
          tunnel: w1036 -> [_ w1093]
          tunnel: [u8 0 w1090] -> w1035
          frame False {
          }
          frame True {
            n608 = Split Number(x=w1093) -> (hi(x)=w1094:u32, lo(x)=w1095:u32)
            n609 = Split Number(x=w1094) -> (lo(x)=w1096:u16)  [unwired: 1 out]
            n610 = Split Number(x=w1095) -> (hi(x)=w1097:u16, lo(x)=w1098:u16)
            n611 = Build Array "BD 1 nu Stack"(w1096, w1097, w1098) -> (w1092:u16[])
            n612 = for {
              tunnel: w1092 -> [w1105] mode=indexing
              shift-right: [w1101] -> w1090
              shift-left: u8 0 -> [w1102]
              n613 = xnode ("FIFO Method Node")("Element"=w1105, "Timeout"="Trap FIFO Set Timeout") -> ("Timed Out?"=w1104:bool)  [unwired: 1 in, 1 out]
              n614 = Boolean To (0,1)(Boolean=w1104) -> (0, 1=w1103:i16)
              n615 = To Unsigned Byte Integer(number=w1103) -> (unsigned 8bit integer=w1100:u8)
              n616 = Add(x=w1100, y=w1102) -> (x+y=w1101:u8)
            }
          }
        }
        n617 = To Unsigned Word Integer(number=w1035) -> (unsigned 16bit integer=w1034:u16)
        n618 = feedback #50(u16 0) -> (w1048:u16)
        n619 = Add(x=w1034, y=w1048) -> (x+y=w1047:u16)
        "Trap Pos FIFO Timeout" <- w1047
        n620 = feedback-in #50(w1047) -> ()
        n621 = feedback-in #51(w1071) -> ()
        n622 = feedback #51(w1071) -> (w1070:u16)
        n623 = Subtract(x=w1071, y=w1070) -> (x-y=w1069:u16)
        n624 = xnode "FPGA I/O Node"("Connector1/DIO31"=FALSE ("Connector1/DIO34")) -> ()  [unwired: 1 in, 1 out]
        n625 = Subtract(x=w1069, y=w1068) -> (x-y=w1039:u16)
        n626 = Boolean To (0,1)(Boolean="+ phase") -> (0, 1=w1064:i16)
        n627 = Multiply(x=w1064, y="Phase count adjustment") -> (x*y=w1058:i16)
        n628 = Subtract(x="ai count", y=w1039) -> (x-y=w1062:u16)
        n629 = Number To Boolean Array(number=w1039) -> (Boolean array=w1040:bool[])
        n630 = feedback #52(i16 0) -> (w1060:i16)
        n631 = Add(x=w1062, y=w1058) -> (x+y=w1061:u16)
        n632 = Subtract(x=w1060, y=w1058) -> (x-y=w1059:i16)
        "Relative phase" <- w1059
        n633 = feedback-in #52(w1059) -> ()
        n634 = Or Array Elements(Boolean array=w1040) -> (logical OR=w1038:bool)
        n635 = Boolean To (0,1)(Boolean=w1038) -> (0, 1=w1045:i16)
        n636 = To Unsigned Byte Integer(number=w1045) -> (unsigned 8bit integer=w1042:u8)
        n637 = feedback #53(u8 0) -> (w1043:u8)
        n638 = Add(x=w1042, y=w1043) -> (x+y=w1041:u8)
        "AI Late Counter" <- w1041
        n639 = feedback-in #53(w1041) -> ()
      }
    }
  }
  n640 = node-c288(w7) -> ()
  n641 = while "APD 3 Counter" {
    tunnel: w1 -> [_]
    stop <- FALSE stop-if-true
    n642 = flat-sequence {
      frame #0 {
        n643 = xnode "FPGA I/O Method Node"("FPGA I/O In"=refnum<k21> "Connector0/DIO2" ("APD 2 DO"), "Timeout"=-1) -> ()  [unwired: 2 out]
      }
      frame #1 {
        n644 = local read "APD3 int gate"() -> (w1147:bool)
        n645 = case shown="True" w1147 {
          frame False {
          }
          frame True {
            n646 = local read "APD3 out state"() -> (w1148:bool)
            n647 = case shown="True" w1148 {
              frame False {
                n648 = local read "APD 3 Counts 0"() -> (w1150:u32)
                n649 = Increment(x=w1150) -> (x+1=→"APD 3 Counts 0":u32)
              }
              frame True {
                n650 = local read "APD 3 Counts 1"() -> (w1152:u32)
                n651 = Increment(x=w1152) -> (x+1=→"APD 3 Counts 1":u32)
              }
            }
          }
        }
      }
    }
  }
  n652 = while "APD 3 Gating" {
    shift-right: [w1156] -> _
    shift-left: w1 -> [w1161]
    shift-right: [w1155] -> _
    shift-left: w5 -> [w1153]
    stop <- FALSE stop-if-true
    n653 = flat-sequence {
      tunnel: w1161 -> [w1164]
      tunnel: [w1165] -> w1159
      tunnel: [w1164] -> w1157
      tunnel: [w1163] -> w1154
      tunnel: w1153 -> [w1163]
      tunnel: [w1168] -> w1160
      tunnel: w1159 -> [w1168]
      tunnel: [w1167] -> w1158
      tunnel: w1157 -> [w1167]
      tunnel: w1154 -> [w1166]
      tunnel: [w1189] -> w1156
      tunnel: w1160 -> [w1200]
      tunnel: w1158 -> [w1197]
      tunnel: [w1169] -> w1155
      frame #0 {
        n654 = call "Loop Timer15"("Count(Ticks)"=w1164) -> ("Tick Count(Ticks)"=w1165:u16)
      }
      frame #1 {
        # "Signal maybe then sent through \na transistor before APD"
        n655 = xnode "FPGA I/O Node"("Connector0/DIO12"=w1166, "Connector0/DIO13"=w1166, "Connector0/DIO14"=w1166, "Connector0/DIO15"=w1166) -> ()  [unwired: 4 in, 4 out]
        "APD3 int gate" <- w1166
      }
      frame #2 {
        n656 = local read "APD Gate OFF Count"() -> (w1174:u16)
        n657 = local read "APD Gate ON Count"() -> (w1175:u16)
        n658 = feedback #54(TRUE) -> (w1194:bool)
        n659 = feedback-in #55(w1200) -> ()
        n660 = feedback #55(w1200) -> (w1199:u16)
        n661 = Not(x=w1194) -> (.not. x?=w1192:bool)
        n662 = feedback-in #54(w1192) -> ()
        n663 = Subtract(x=w1200, y=w1199) -> (x-y=w1198:u16)
        n664 = Select(t=w1175, s=w1192, f=w1174) -> (s? t:f=w1196:u16)
        n665 = Subtract(x=w1198, y=w1197) -> (x-y=w1177:u16)
        n666 = Subtract(x=w1196, y=w1177) -> (x-y=w1188:u16)
        n667 = Number To Boolean Array(number=w1177) -> (Boolean array=w1178:bool[])
        n668 = Or Array Elements(Boolean array=w1178) -> (logical OR=w1176:bool)
        n669 = Boolean To (0,1)(Boolean=w1176) -> (0, 1=w1183:i16)
        n670 = Boolean To (0,1)(Boolean="+ phase (APD 3 Gate)") -> (0, 1=w1186:i16)
        n671 = To Unsigned Byte Integer(number=w1183) -> (unsigned 8bit integer=w1180:u8)
        n672 = Multiply(x=w1186, y="Phase count adjustment (APD 3 Gate)") -> (x*y=w1184:i16)
        n673 = feedback #56(u8 0) -> (w1181:u8)
        n674 = Add(x=w1180, y=w1181) -> (x+y=w1179:u8)
        "APD 3 Gate Late Counter" <- w1179
        n675 = feedback-in #56(w1179) -> ()
        n676 = Add(x=w1188, y=w1184) -> (x+y=w1189:u16)
        n677 = feedback #57(i16 0) -> (w1191:i16)
        n678 = Subtract(x=w1191, y=w1184) -> (x-y=w1190:i16)
        "APD 3 Gate Relative Phase" <- w1190
        n679 = feedback-in #57(w1190) -> ()
        n680 = local read "APD Gate Operating Mode"() -> (w1173:u8)
        n681 = case shown="2" w1173 {
          tunnel: [TRUE FALSE w1203] -> w1170
          tunnel: w1194 -> [_ _ w1203]
          frame 0, Default {
          }
          frame 1 {
          }
          frame 2 {
          }
        }
        n682 = local read "Invert APD Gate"() -> (w1172:bool)
        n683 = Not(x=w1170) -> (.not. x?=w1171:bool)
        n684 = Select(t=w1171, s=w1172, f=w1170) -> (s? t:f=w1169:bool)
      }
    }
  }
  n685 = while "633 nm red  fluorescent laser interlacing (DO to IA 633 nm AOM ME amp)." {
    shift-right: [w1207] -> _
    shift-left: w1 -> [w1212]
    shift-right: [w1206] -> _
    shift-left: w2 -> [w1204]
    stop <- FALSE stop-if-true
    n686 = flat-sequence {
      tunnel: w1212 -> [w1215]
      tunnel: [w1216] -> w1210
      tunnel: [w1215] -> w1208
      tunnel: [w1214] -> w1205
      tunnel: w1204 -> [w1214]
      tunnel: [w1219] -> w1211
      tunnel: w1210 -> [w1219]
      tunnel: [w1218] -> w1209
      tunnel: w1208 -> [w1218]
      tunnel: w1205 -> [w1217]
      tunnel: [w1228] -> w1207
      tunnel: w1211 -> [w1248]
      tunnel: w1209 -> [w1245]
      tunnel: [w1237] -> w1206
      frame #0 {
        n687 = call "Loop Timer11"("Count(Ticks)"=w1215) -> ("Tick Count(Ticks)"=w1216:u16)
      }
      frame #1 {
        # "Then to PRL 440 amp"
        n688 = xnode "FPGA I/O Node"("Connector1/DIO32"=w1217) -> ()  [unwired: 1 in, 1 out]
      }
      frame #2 {
        n689 = feedback-in #58(w1248) -> ()
        n690 = feedback #58(w1248) -> (w1247:u16)
        n691 = Subtract(x=w1248, y=w1247) -> (x-y=w1246:u16)
        n692 = Subtract(x=w1246, y=w1245) -> (x-y=w1221:u16)
        n693 = Number To Boolean Array(number=w1221) -> (Boolean array=w1222:bool[])
        n694 = Or Array Elements(Boolean array=w1222) -> (logical OR=w1220:bool)
        n695 = Boolean To (0,1)(Boolean="+ phase (RI)") -> (0, 1=w1233:i16)
        n696 = Multiply(x=w1233, y="Phase count adjustment (RI)") -> (x*y=w1230:i16)
        n697 = Boolean To (0,1)(Boolean=w1220) -> (0, 1=w1227:i16)
        n698 = To Unsigned Byte Integer(number=w1227) -> (unsigned 8bit integer=w1224:u8)
        n699 = feedback #59(i16 0) -> (w1231:i16)
        n700 = feedback #60(u8 0) -> (w1225:u8)
        n701 = Add(x=w1224, y=w1225) -> (x+y=w1223:u8)
        "RI Late Counter" <- w1223
        n702 = feedback-in #60(w1223) -> ()
        n703 = Subtract(x=w1231, y=w1230) -> (x-y=w1229:i16)
        "RI Relative phase" <- w1229
        n704 = feedback-in #59(w1229) -> ()
        n705 = feedback #61(TRUE) -> (w1240:bool)
        n706 = case shown="2" "Red Laser Operating Mode" {
          tunnel: [TRUE FALSE w1254] -> w1237
          tunnel: w1240 -> [_ _ w1251]
          frame 0, Default {
          }
          frame 1 {
          }
          frame 2 {
            n707 = Not(x=w1251) -> (.not. x?=w1253:bool)
            n708 = Select(t=w1253, s="Invert RI", f=w1251) -> (s? t:f=w1254:bool)
          }
        }
        n709 = Not(x=w1240) -> (.not. x?=w1236:bool)
        n710 = Select(t="Red interlace ON count", s=w1236, f="Red interlace OFF count") -> (s? t:f=w1242:u16)
        n711 = Subtract(x=w1242, y=w1221) -> (x-y=w1234:u16)
        n712 = Add(x=w1234, y=w1230) -> (x+y=w1228:u16)
        n713 = feedback-in #61(w1236) -> ()
      }
    }
  }
  n714 = while "473 nm blue  fluorescent laser interlacing (DO to blue laser digital control input)." {
    shift-right: [w1258] -> _
    shift-left: w1 -> [w1263]
    shift-right: [w1257] -> _
    shift-left: w2 -> [w1255]
    stop <- FALSE stop-if-true
    n715 = flat-sequence {
      tunnel: w1263 -> [w1266]
      tunnel: [w1267] -> w1261
      tunnel: [w1266] -> w1259
      tunnel: [w1265] -> w1256
      tunnel: w1255 -> [w1265]
      tunnel: [w1270] -> w1262
      tunnel: w1261 -> [w1270]
      tunnel: [w1269] -> w1260
      tunnel: w1259 -> [w1269]
      tunnel: w1256 -> [w1268]
      tunnel: [w1279] -> w1258
      tunnel: w1262 -> [w1299]
      tunnel: w1260 -> [w1296]
      tunnel: [w1288] -> w1257
      frame #0 {
        n716 = call "Loop Timer14"("Count(Ticks)"=w1266) -> ("Tick Count(Ticks)"=w1267:u16)
      }
      frame #1 {
        n717 = xnode "FPGA I/O Node"("Connector1/DIO28"=w1268) -> ()  [unwired: 1 in, 1 out]
      }
      frame #2 {
        n718 = feedback-in #62(w1299) -> ()
        n719 = feedback #62(w1299) -> (w1298:u16)
        n720 = Subtract(x=w1299, y=w1298) -> (x-y=w1297:u16)
        n721 = Subtract(x=w1297, y=w1296) -> (x-y=w1272:u16)
        n722 = Number To Boolean Array(number=w1272) -> (Boolean array=w1273:bool[])
        n723 = Or Array Elements(Boolean array=w1273) -> (logical OR=w1271:bool)
        n724 = Boolean To (0,1)(Boolean="+ phase (BI D)") -> (0, 1=w1284:i16)
        n725 = Multiply(x=w1284, y="Phase count adjustment (BI D)") -> (x*y=w1281:i16)
        n726 = Boolean To (0,1)(Boolean=w1271) -> (0, 1=w1278:i16)
        n727 = To Unsigned Byte Integer(number=w1278) -> (unsigned 8bit integer=w1275:u8)
        n728 = feedback #63(i16 0) -> (w1282:i16)
        n729 = feedback #64(u8 0) -> (w1276:u8)
        n730 = Add(x=w1275, y=w1276) -> (x+y=w1274:u8)
        "Blue Late Counter (D)" <- w1274
        n731 = feedback-in #64(w1274) -> ()
        n732 = Subtract(x=w1282, y=w1281) -> (x-y=w1280:i16)
        "BI Relative phase (D)" <- w1280
        n733 = feedback-in #63(w1280) -> ()
        n734 = feedback #65(TRUE) -> (w1291:bool)
        n735 = case shown="2" "Blue Laser Operating Mode (D)" {
          tunnel: [TRUE FALSE w1305] -> w1288
          tunnel: w1291 -> [_ _ w1302]
          frame 0, Default {
          }
          frame 1 {
          }
          frame 2 {
            n736 = Not(x=w1302) -> (.not. x?=w1304:bool)
            n737 = Select(t=w1304, s="Invert BI (D)", f=w1302) -> (s? t:f=w1305:bool)
          }
        }
        n738 = Not(x=w1291) -> (.not. x?=w1287:bool)
        n739 = Select(t="Blue interlace ON count (D)", s=w1287, f="Blue interlace OFF count (D)") -> (s? t:f=w1293:u16)
        n740 = Subtract(x=w1293, y=w1272) -> (x-y=w1285:u16)
        n741 = Add(x=w1285, y=w1281) -> (x+y=w1279:u16)
        n742 = feedback-in #65(w1287) -> ()
      }
    }
  }
  n743 = while "Blue fluorescent laser interlacing (AO control direct to laser)." {
    shift-right: [w1311] -> _
    shift-left: w1 -> [w1314]
    shift-right: [w1308] -> _
    shift-left: i16 0 -> [w1306]
    stop <- FALSE stop-if-true
    n744 = flat-sequence {
      tunnel: w1314 -> [w1317]
      tunnel: [w1318] -> w1313
      tunnel: [w1317] -> w1312
      tunnel: [w1316] -> w1307
      tunnel: w1306 -> [w1316]
      tunnel: [w1321] -> w1310
      tunnel: w1313 -> [w1321]
      tunnel: [w1320] -> w1309
      tunnel: w1312 -> [w1320]
      tunnel: w1307 -> [w1319]
      tunnel: [w1331] -> w1311
      tunnel: [w1347] -> w1308
      tunnel: w1310 -> [w1359]
      tunnel: w1309 -> [w1356]
      frame #0 {
        n745 = call "Loop Timer13"("Count(Ticks)"=w1317) -> ("Tick Count(Ticks)"=w1318:u16)
      }
      frame #1 {
        n746 = xnode "FPGA I/O Node"("Connector0/AO3"=w1319) -> ()  [unwired: 1 in, 1 out]
      }
      frame #2 {
        n747 = Subtract(x="Blue OFF count (AO)", y="Blue current ON count adj (AO)") -> (x-y=w1340:u16)
        n748 = feedback-in #66(w1359) -> ()
        n749 = feedback #66(w1359) -> (w1358:u16)
        n750 = Add(x="Blue current ON count adj (AO)", y="Blue ON count (AO)") -> (x+y=w1341:u16)
        n751 = Subtract(x=w1359, y=w1358) -> (x-y=w1357:u16)
        n752 = Subtract(x=w1357, y=w1356) -> (x-y=w1324:u16)
        n753 = Number To Boolean Array(number=w1324) -> (Boolean array=w1325:bool[])
        n754 = Boolean To (0,1)(Boolean="+ phase (BI AO)") -> (0, 1=w1337:i16)
        n755 = Or Array Elements(Boolean array=w1325) -> (logical OR=w1323:bool)
        n756 = Boolean To (0,1)(Boolean=w1323) -> (0, 1=w1330:i16)
        n757 = Multiply(x=w1337, y="Phase count adjustment (BI AO)") -> (x*y=w1333:i16)
        n758 = To Unsigned Byte Integer(number=w1330) -> (unsigned 8bit integer=w1326:u8)
        n759 = feedback #67(u8 0) -> (w1328:u8)
        n760 = Add(x=w1326, y=w1328) -> (x+y=w1327:u8)
        "BI Late Counter (AO)" <- w1327
        n761 = feedback-in #67(w1327) -> ()
        n762 = feedback #68(i16 0) -> (w1334:i16)
        n763 = Subtract(x=w1334, y=w1333) -> (x-y=w1332:i16)
        "BI Relative phase (AO)" <- w1332
        n764 = feedback-in #68(w1332) -> ()
        n765 = feedback #69(TRUE) -> (w1351:bool)
        n766 = case shown="2" "BI Operating Mode (AO)" {
          tunnel: [TRUE FALSE w1375] -> w1342
          tunnel: w1351 -> [_ _ w1372]
          frame 0, Default {
          }
          frame 1 {
          }
          frame 2 {
            n767 = Not(x=w1372) -> (.not. x?=w1374:bool)
            n768 = Select(t=w1374, s="Invert BI (AO)", f=w1372) -> (s? t:f=w1375:bool)
          }
        }
        n769 = And(x=w1342, y="Blue FB On/Off") -> (x .and. y?=w1343:bool)
        n770 = case shown="True" w1343 {
          tunnel: "BI Current Out" -> [w1360 _]
          tunnel: [w1360 w1362] -> w1346
          frame False {
          }
          frame True {
            n771 = local read "Blue Intensity"() -> (w1361:i16)
            n772 = Bundle("P5"="P5", "I5"="I5", "D5"="D5") -> (w1363:cluster{"P5":i16, "I5":i16, "D5":i16})  [unwired: 1 in]
            n773 = call "Slower PID.vi"("process variable"=w1361, "reset?"="Blue FB Reset", "setpoint"="Blue FB Setpoint", "PID gains (x 2^8)"=w1363, "output range"=cluster{"output high":i16, "output low":i16} {"output high"=32767, "output low"=0} ("Green FB output range")) -> ("output"=w1362:i16)  [unwired: 10 out]
          }
        }
        n774 = Not(x=w1351) -> (.not. x?=w1348:bool)
        n775 = Select(t=w1341, s=w1348, f=w1340) -> (s? t:f=w1353:u16)
        n776 = Subtract(x=w1353, y=w1324) -> (x-y=w1335:u16)
        n777 = Add(x=w1335, y=w1333) -> (x+y=w1331:u16)
        n778 = feedback-in #69(w1348) -> ()
        n779 = Boolean To (0,1)(Boolean=w1342) -> (0, 1=w1322:i16)
        n780 = Multiply(x=w1322, y=w1346) -> (x*y=w1347:i16)
      }
    }
  }
